vi "SISE-Monitor100-Demo.vi"() -> ()   [LabVIEW 2024]
uses:
  SubVIs-SISE-Monitor100/Control-IonFlux.ctl
  <vilib>/DAQmx/create/channels.llb/DAQmx Create Channel (AI-Voltage-Basic).vi
  <vilib>/Instr/_visa.llb/VISA Configure Serial Port (Instr).vi
  <vilib>/Analysis/NI_AALPro.lvlib
  <vilib>/DAQmx/read.llb/DAQmx Read (Analog 2D DBL NChan NSamp).vi
panel:
  out "Lesepuffer":string
  out "Registerkarte":enum32{"Start", "Record", "Stop"}(tab)
  out "Output V ch 2":bool
  in  "V channel 2":bool
  out "Output V ch 1":bool
  in  "V channel 1":bool
  out "SISE channel 1":bool
  out "Output SISE ch 2":bool
  in  "SISE channel 2":bool
  out "slow":bool
  in  "Scan angle (degrees)":dbl(slide) scale=0.0..90.0
  out "?":dbl
  in  "VISA res. name":refnum<visa-resource-name> caption="VISA-Ressourcenname"
  in  "Start measurement":bool
  out "Data File":bool
  out "Ind. Channel In":bool
  in  "Data file":path
  out "Ind. Channel Out":bool
  out "?":dbl
  out "Record period (round at 5s)":dbl
  in  "Scan distance (µm)":dbl(slide)=50.0 scale=0.0..100.0
  in  "Record period (single track, s)":dbl(slide)=10.112359550561797 scale=0.0..60.0 scale format="%#_2f"
  in  "Manipulator Speed":bool
  out "fast":bool
  in  "Channels In":tag
  in  "Position of manipulator":bool
  out "left":bool
  out "right":bool
  in  "TC 3":T1(tab)
  in  "Range limit\nS1.1 (mV)":dbl(slide)=200.0 min=0.0 max=600.0 scale=0.2..600.0
  in  "Base line\nS1.1 (mV)":dbl(slide) scale=-300.0..300.0
  in  "Range limit\nS1.2 mV":dbl(slide)=30.0 scale=0.1..30.0
  in  "Base line \nS1.2 (mV)":dbl(slide) scale=-15.0..15.0
  out "dV-SISE channel 1":cluster{dbl[], dbl[]}[](graph)
  out "V-SISE channel 1":cluster{dbl[], dbl[]}[](graph)
  out "V-SISE channel 2":cluster{dbl[], dbl[]}[](graph)
  out "dV-SISE channel 2":cluster{dbl[], dbl[]}[](graph)
  in  "Range limit\nS2.1 (mV)":dbl(slide)=200.0 min=0.0 max=600.0 scale=0.2..600.0
  in  "Base line\nS2.1 (mV)":dbl(slide) scale=-300.0..300.0
  in  "Base line \nS2.2 (mV)":dbl(slide) scale=-15.0..15.0
  in  "Range limit\nS2.2 (mV)":dbl(slide)=30.0 scale=0.1..30.0
  out "Voltage channel 1":cluster{dbl[], dbl[]}[](graph)
  in  "Base line\nV1 (V)":dbl(slide) scale=-300.0..300.0
  in  "Range limit\nV1 (V)":dbl(slide)=200.0 min=0.0 max=600.0 scale=0.2..600.0
  in  "Base line\nV2 (V)":dbl(slide) scale=-300.0..300.0
  in  "Range limit\nV2 (V)":dbl(slide)=200.0 min=0.0 max=600.0 scale=0.2..600.0
  out "Voltage channel 2":cluster{dbl[], dbl[]}[](graph)
  out "V channel #2":bool
  out "V channel #1":bool
  out "SISE channel #2":bool
  out "SISE channel #1":bool
  in  "?":T2(tab)
  in  "V SISE\nch #1":dbl(slide)=4.96774193548387 scale=-10.0..10.0
  out "Vprobe SISE 1":cluster{dbl[], dbl[]}[](graph)
  in  "V SISE\nch #2":dbl(slide)=4.96774193548387 scale=-10.0..10.0
  out "Vprobe SISE 2":cluster{dbl[], dbl[]}[](graph)
  in  "Vch #1":dbl(slide)=5.096774193548386 scale=-10.0..10.0
  out "Vprobe V 1":cluster{dbl[], dbl[]}[](graph)
  in  "Vch\n#2":dbl(slide)=5.096774193548386 scale=-10.0..10.0
  out "Vprobe V 2":cluster{dbl[], dbl[]}[](graph)
  in  "Enable change position 0":bool
  out "Raw data file":path
  in  "Stop measurent":bool
  out "Position probe":cluster{dbl[], dbl[]}[](graph)
  in  "Add Mark":bool
  in  "Event Mark":string
  out "Stop recording":bool
  out "String":string
  out "E-mark on":T3
  out "?":string
  in  "Bildlaufleiste":i32(c297)
  in  "Start fit (% of rec. period)":dbl(slide)=50.0 scale=0.0..100.0
  in  "?":enum32{"dV SISE 1", "dV SISE 2"}(tab)
  out "deltaV SISE 1":cluster{dbl[], "Best Linear Fit":dbl[]}[](graph)
  out "deltaV SISE 2":cluster{dbl[], "Best Linear Fit":dbl[]}[](graph)
  in  "Zoom from start":dbl(slide) scale=0.0..100.0
  in  "Zoom from end":dbl(slide)=100.0 scale=0.0..100.0
  in  "Stop programm":bool
  in  "New measurement":bool
  out "Stop recording 2":bool
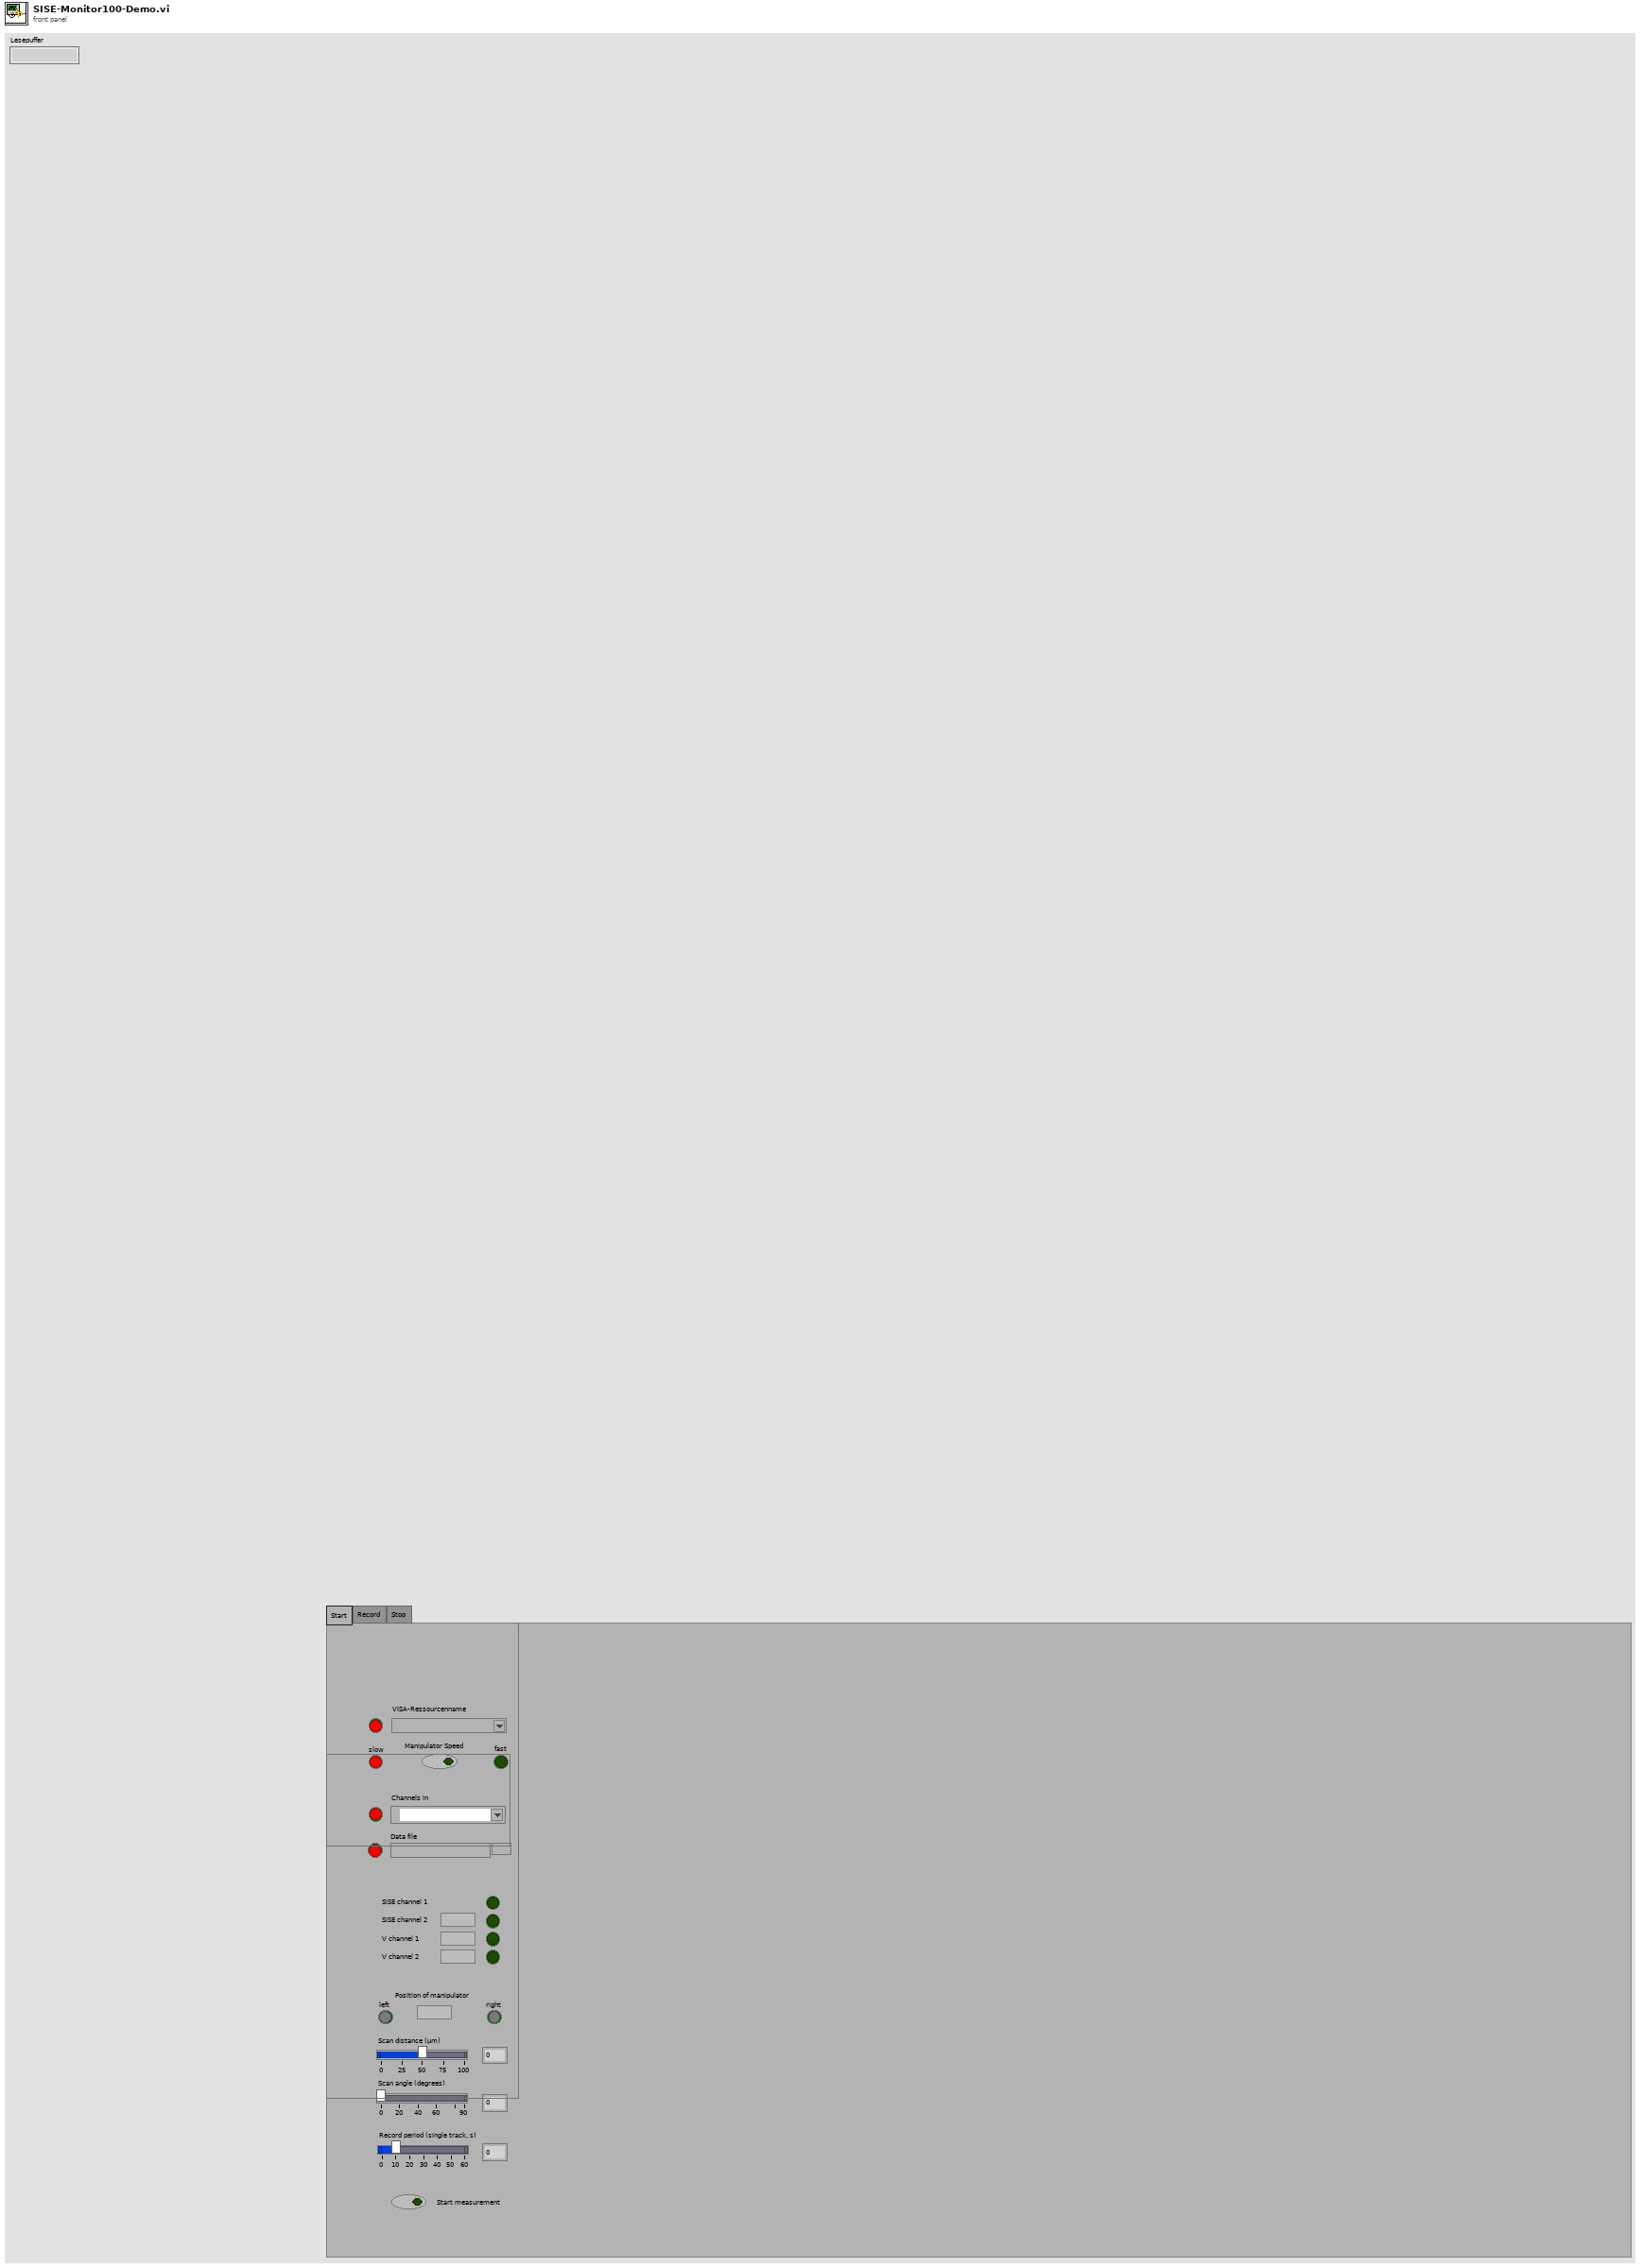
[diagram p1: front panel]
types:
  T1 = enum32{"SISE channel #1", "SISE channel #2", "V channel #1", "V channel #2"}
  T2 = enum32{"SISE chan #1", "SISE chan #2", "V chan #1", "V chan #2"}
  T3 = typedef "Control-IonFlux.ctl" = bool
  T4 = cluster{"refnum out":refnum<file>, "status":bool, "code":i32, "source":string}
  T5 = cluster{"task out":refnum<k21>, "status":bool, "code":i32, "source":string}
  T6 = enum16{"open", "replace", "create", "open or create", "replace or create", "replace or create with confirmation"}
  T7 = cluster{"refnum":refnum<file>, "status":bool, "code":i32, "source":string}
  T8 = cluster{dbl[], dbl[], "Best Linear Fit":dbl[], dbl[], dbl[]}
  T9 = cluster{"Array (Ausgang)":dbl[], "Array (Ausgang)":dbl[]}
  T10 = cluster{"Array (Ausgang)":dbl[], "Array (Ausgang)":dbl[]}[]
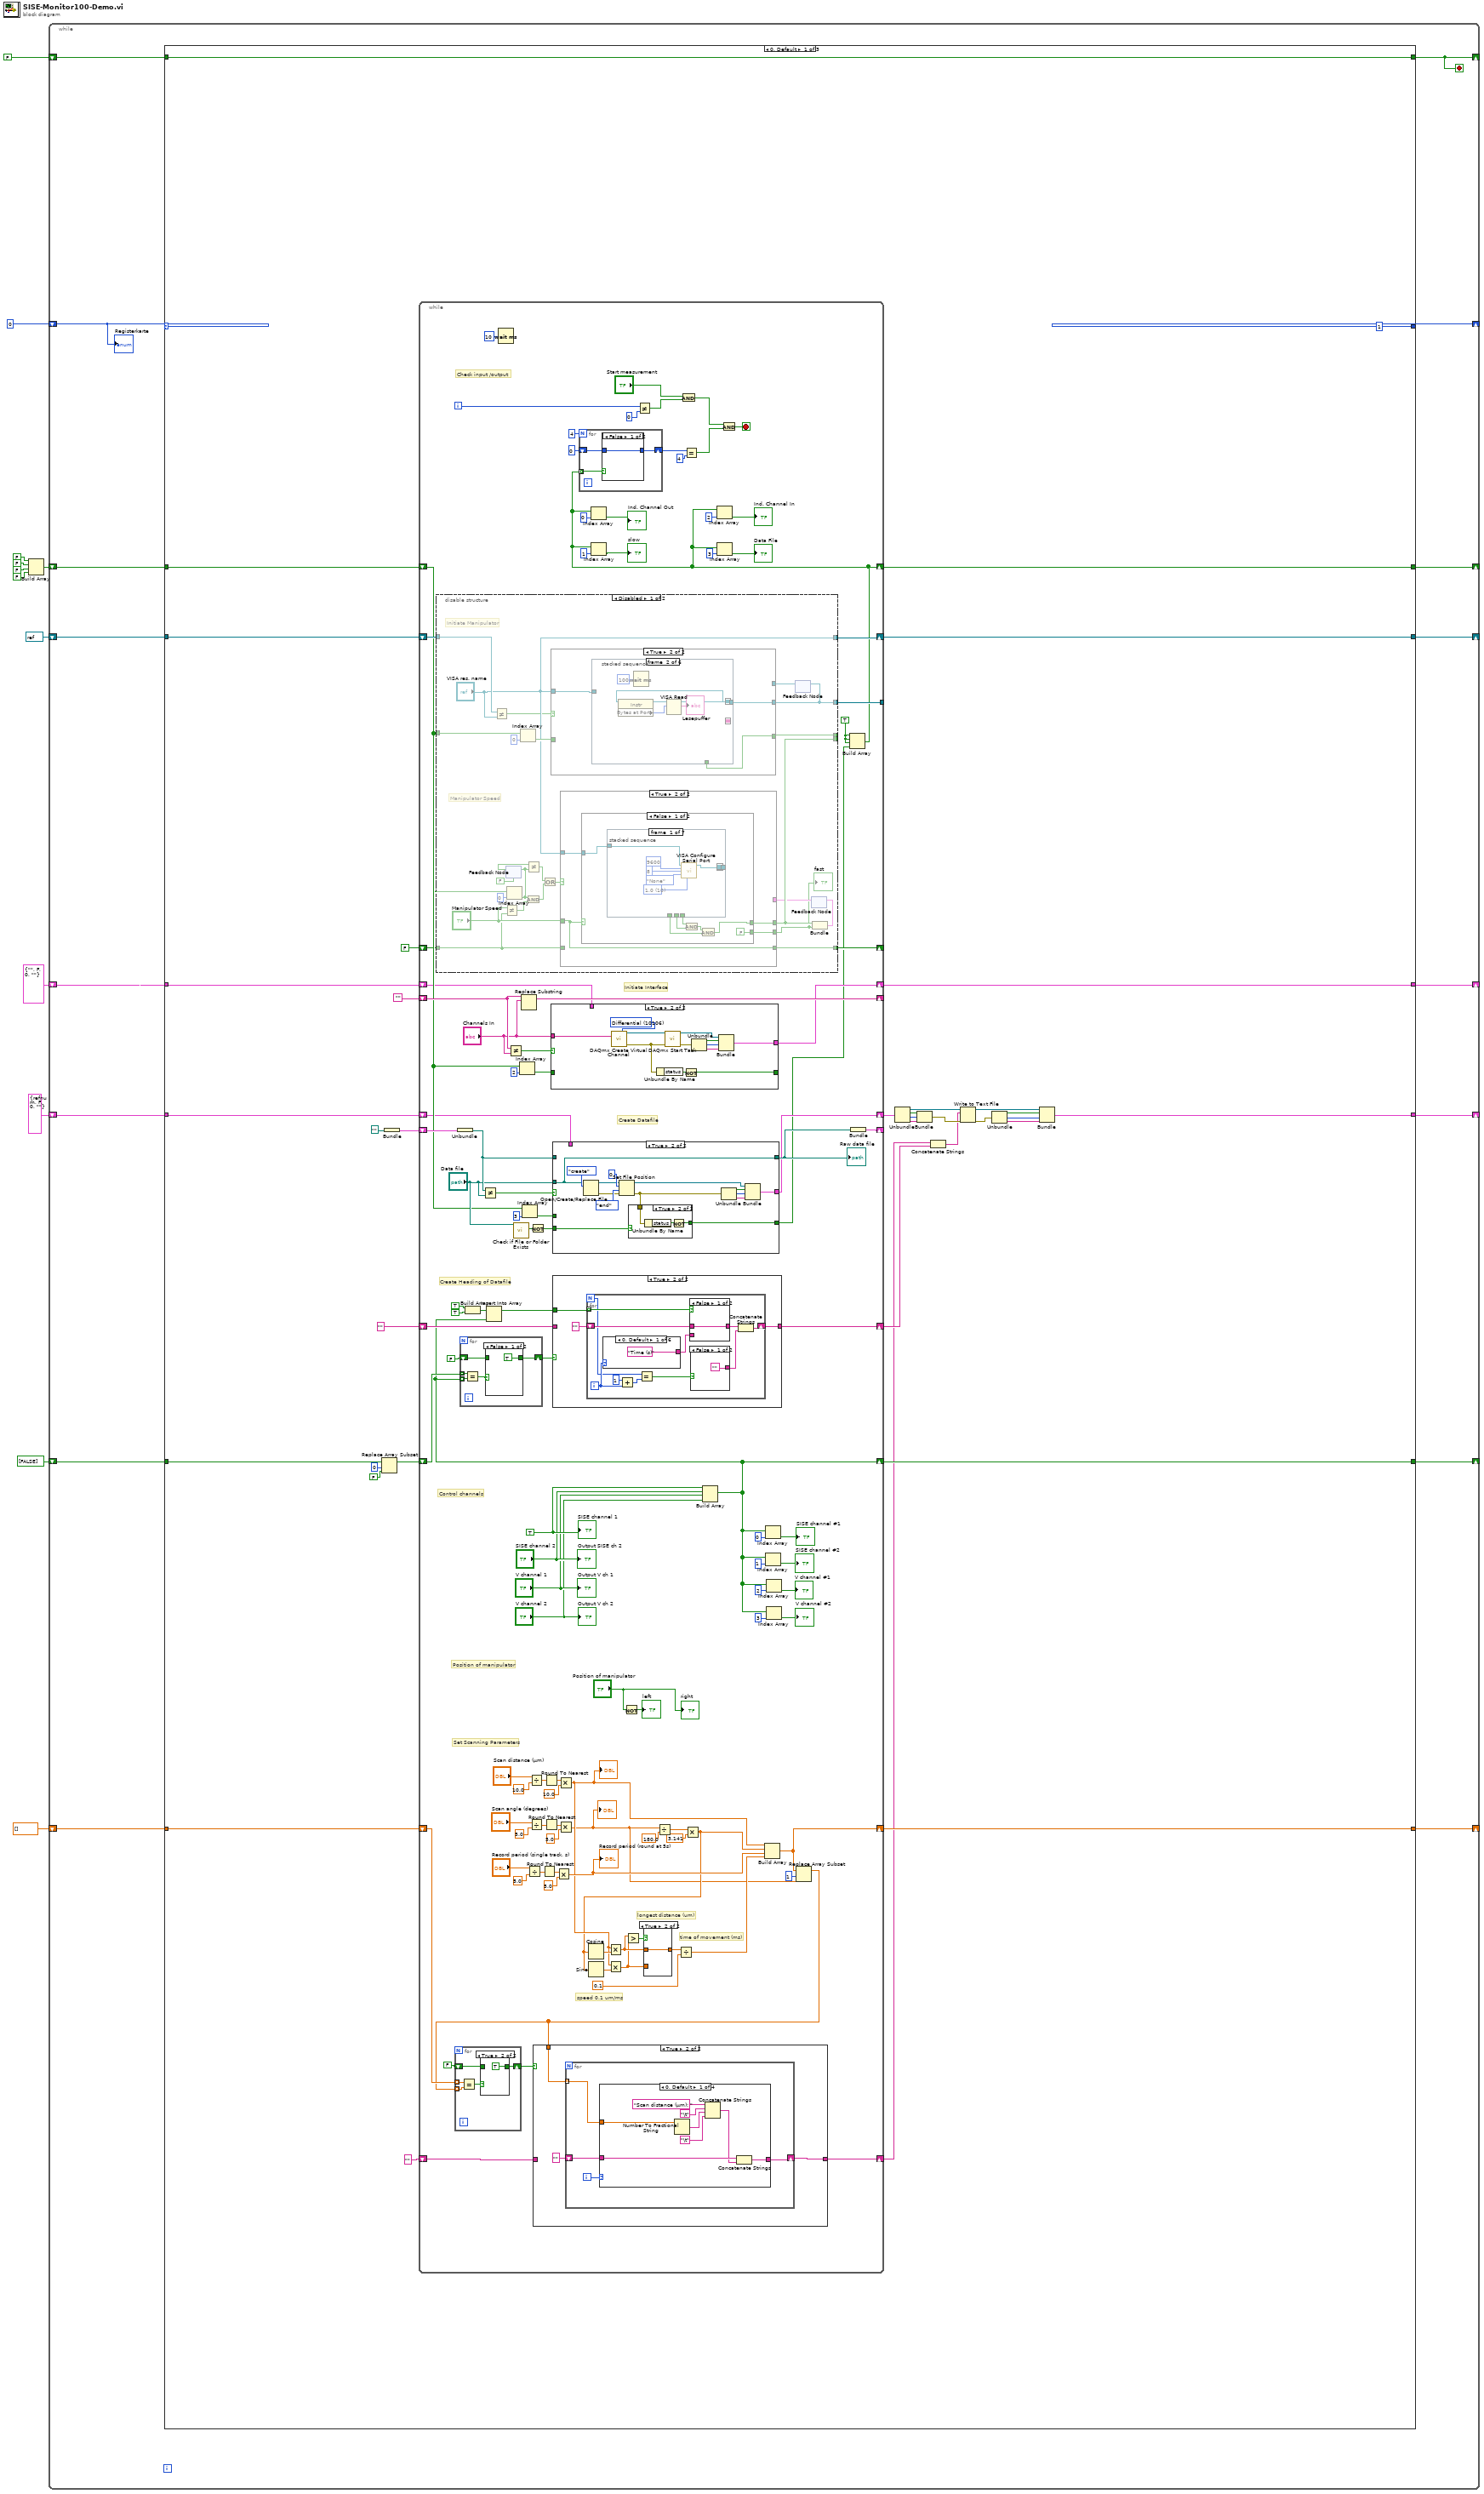
[diagram p0: block diagram]
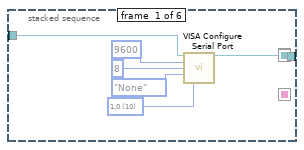
[diagram p3: hidden frame]
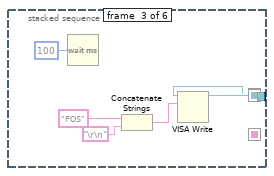
[diagram p4: hidden frame]
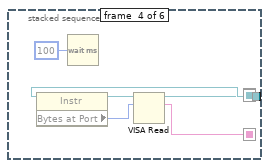
[diagram p5: hidden frame]
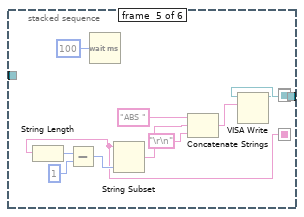
[diagram p6: hidden frame]
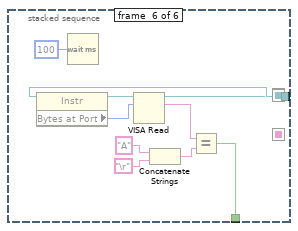
[diagram p7: hidden frame]
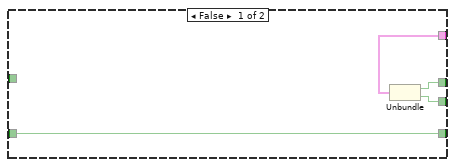
[diagram p8: hidden frame]
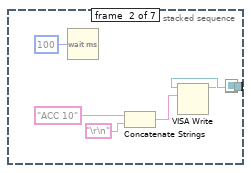
[diagram p9: hidden frame]
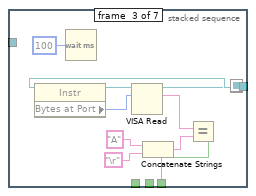
[diagram p10: hidden frame]
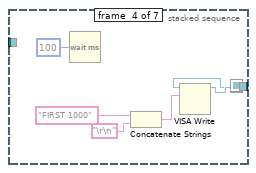
[diagram p11: hidden frame]
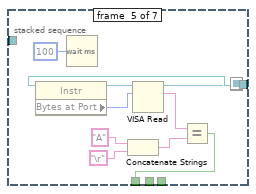
[diagram p12: hidden frame]
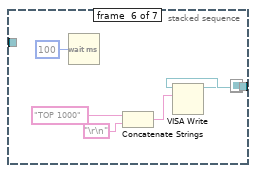
[diagram p13: hidden frame]
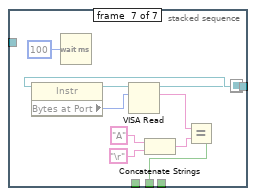
[diagram p14: hidden frame]
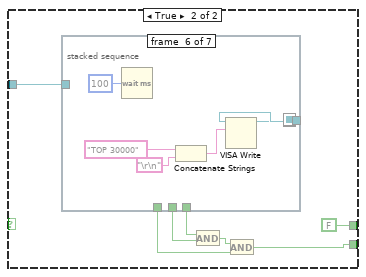
[diagram p15: hidden frame]
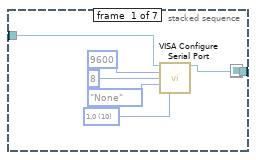
[diagram p16: hidden frame]
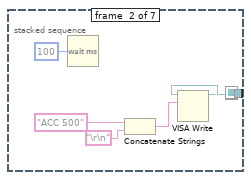
[diagram p17: hidden frame]
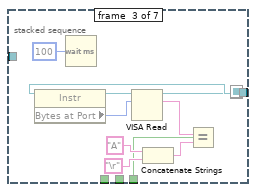
[diagram p18: hidden frame]
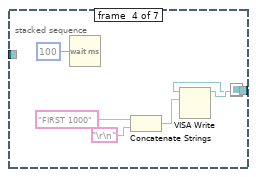
[diagram p19: hidden frame]
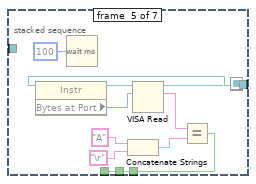
[diagram p20: hidden frame]
diagram:
  n1 = Build Array(FALSE, FALSE, FALSE, FALSE) -> (w1:bool[])
  n2 = while {
    shift-right: [w28] -> _
    shift-left: 0 -> [w27]
    shift-right: [w25] -> _
    shift-left: refnum<visa-resource-name> refnum ("VISA res. name") -> [w26]
    shift-right: [w23] -> _
    shift-left: T5 {"task out"="", "status"=FALSE, "code"=0, "source"=""} -> [w24]
    shift-right: [w19] -> _
    shift-left: T4 {"refnum out"=refnum, "status"=FALSE, "code"=0, "source"=""} -> [w20]
    shift-right: [w22] -> _
    shift-left: dbl[] [] -> [w21]
    shift-right: [w18] -> _
    shift-left: bool[] [FALSE] -> [w17]
    shift-right: [w15] -> _
    shift-left: FALSE -> [w16]
    shift-right: [w13] -> _
    shift-left: w1 -> [w14]
    stop <- w15 stop-if-true
    n3 = case shown="0, Default" w27 {
      tunnel: [1 2 0] -> w28
      tunnel: w26 -> [w60 w559 w1622]
      tunnel: [w59 w558 w1622] -> w25
      tunnel: w24 -> [w58 w557 w1621]
      tunnel: [w57 w553 w1621] -> w23
      tunnel: [w40 w532 w1619] -> w19
      tunnel: w20 -> [w56 w536 w1619]
      tunnel: [w55 w546 w1620] -> w22
      tunnel: w21 -> [w54 w546 w1620]
      tunnel: w17 -> [w31 w522 w1618]
      tunnel: [w53 w529 w1618] -> w18
      tunnel: w16 -> [w39 w521 w1617]
      tunnel: [w39 w521 w1616] -> w15
      tunnel: w14 -> [w33 w520 w1615]
      tunnel: [w38 w520 w1615] -> w13
      frame 0, Default {
        n4 = Replace Array Subset(array=w31, new element=FALSE ("Neues Element/Teil-Array"), index=0 ("Index")) -> (w32:bool[])
        n5 = Bundle(path "") -> (w61:cluster{path})  [unwired: 1 in]
        n6 = while {
          shift-right: [w117] -> w59
          shift-left: w60 -> [w165]
          shift-right: [w90] -> w38
          shift-left: w33 -> [w123]
          tunnel: [w124] -> _
          shift-right: [w160] -> _
          shift-left: "" -> [w159]
          shift-right: [w151] -> _
          shift-left: w61 -> [w153]
          shift-right: [w118] -> _
          shift-left: FALSE -> [w122]
          shift-right: [w115] -> w57
          shift-left: w58 -> [w116]
          shift-right: [w113] -> w51
          shift-left: w56 -> [w112]
          shift-right: [w73] -> w55
          shift-left: w54 -> [w77]
          shift-right: [w82] -> w53
          shift-left: w32 -> [w85]
          shift-right: [w87] -> w36
          shift-left: "" -> [w86]
          shift-right: [w79] -> w35
          shift-left: "" -> [w75]
          i -> [w80]
          stop <- w83 stop-if-true
          w68 = TRUE
          w108 = TRUE
          # "Position of manipulator"
          # "Set Scanning Parameters"
          # "Control channels"
          # "Create Heading of Datafile"
          # "Create Datafile"
          # "Initiate Interface"
          # "Check input /output"
          # "speed 0.1 um/ms"
          # "longest distance (um)"
          # "time of movement (ms)"
          n7 = disable-structure shown="Disabled" {
            disable-tunnel: w165 -> [w200 _]
            disable-tunnel: [w196 _] -> w124
            disable-tunnel: w123 -> [w194 _]
            disable-tunnel: w122 -> [w191 _]
            disable-tunnel: [w184 _] -> _
            disable-tunnel: [w183 _] -> _
            disable-tunnel: [w180 _] -> w118
            disable-tunnel: ["VISA res. name" _] -> w117
            frame Disabled {
              # "Manipulator Speed"
              # "Initiate Manipulator"
              n8 = Not Equal?(x=w200, y="VISA res. name") -> (x != y?=w177:bool)
              n9 = Not Equal?(x="Manipulator Speed", y=w191) -> (x != y?=w193:bool)
              n10 = feedback #1(FALSE) -> (w188:bool)
              n11 = Index Array(array=w194, index=0 ("Index")) -> (element=w189:bool)
              n12 = feedback-in #1(w189) -> ()
              n13 = Index Array(array=w194, index=0 ("Index")) -> (element=w198:bool)
              n14 = Not Equal?(x=w188, y=w189) -> (x != y?=w187:bool)
              n15 = And(x=w189, y=w193) -> (x .and. y?=w185:bool)
              n16 = Or(x=w187, y=w185) -> (x .or. y?=w186:bool)
              n17 = feedback #2() -> (w197:refnum<visa-resource-name>)  [unwired: 1 in]
              n18 = case shown="True" w177 {
                tunnel: w198 -> [w202 _]
                tunnel: [w202 w205] -> w184
                tunnel: "VISA res. name" -> [_ w204]
                tunnel: [w201 w203] -> w196
                tunnel: w197 -> [w201 _]
                frame False {
                }
                frame True {
                  n19 = stacked-sequence {
                    seq-local: [w206 _ _ _ _ _] -> [_ w213 _ _ _ _]
                    seq-local: [_ w214 _ _ _ _] -> [_ _ w218 _ _ _]
                    seq-local: [_ _ w219 _ _ _] -> [_ _ _ w226 _ _]
                    seq-local: [_ _ _ w225 _ _] -> [_ _ _ _ w237 _]
                    seq-local: [_ _ _ w224 _ _] -> [_ _ _ _ w231 _]
                    seq-local: [_ _ _ _ w236 _] -> [_ _ _ _ _ w247]
                    tunnel: w204 -> [w211 _ _ _ _ _]
                    tunnel: [_ _ _ _ _ w246] -> w203
                    tunnel: [_ _ _ _ _ w241] -> w205
                    frame #0 {
                      w207 = u16 10 items=["1,0"=10, "1,5"=15, "2,0"=20] ("stop bits (10: 1 bit)")
                      n20 = call-poly "VISA Configure Serial Port"("VISA resource name"=w211, "baud rate (9600)"=u32 9600, "data bits (8)"=u16 8, "parity (0:none)"=enum16{"None", "Odd", "Even", "Mark", "Space"}."None", "stop bits (10: 1 bit)"=w207) -> ("VISA resource name out"=w206:refnum<visa-resource-name>)  [unwired: 9 in, 1 out]
                    }
                    frame #1 {
                      n21 = property class="Instr"(reference=w213) -> (reference out=w216:refnum<visa-resource-name>, "Bytes at Port"=w215:u32)  [unwired: 1 in, 1 out]
                      n22 = Wait (ms)(milliseconds to wait=u32 100) -> ()  [unwired: 1 out]
                      n23 = VISA Read(VISA resource name=w216, byte count=w215) -> (VISA resource name out=w214:refnum<visa-resource-name>, read buffer=→"Lesepuffer":string)  [unwired: 1 in, 2 out]
                    }
                    frame #2 {
                      n24 = Wait (ms)(milliseconds to wait=u32 100) -> ()  [unwired: 1 out]
                      n25 = Concatenate Strings("POS", "\r\n") -> (w220:string)
                      n26 = VISA Write(VISA resource name=w218, write buffer=w220) -> (VISA resource name out=w219:refnum<visa-resource-name>)  [unwired: 1 in, 2 out]
                    }
                    frame #3 {
                      n27 = property class="Instr"(reference=w226) -> (reference out=w227:refnum<visa-resource-name>, "Bytes at Port"=w228:u32)  [unwired: 1 in, 1 out]
                      n28 = Wait (ms)(milliseconds to wait=u32 100) -> ()  [unwired: 1 out]
                      n29 = VISA Read(VISA resource name=w227, byte count=w228) -> (VISA resource name out=w225:refnum<visa-resource-name>, read buffer=w224:string)  [unwired: 1 in, 2 out]
                    }
                    frame #4 {
                      n30 = String Length(string=w231) -> (length=w234:i32)
                      n31 = Subtract(x=w234, y=1) -> (x-y=w232:i32)
                      n32 = Wait (ms)(milliseconds to wait=u32 100) -> ()  [unwired: 1 out]
                      n33 = String Subset(string=w231, length (rest)=w232) -> (substring=w230:string)  [unwired: 1 in]
                      n34 = Concatenate Strings("ABS ", w230, "\r\n") -> (w238:string)
                      n35 = VISA Write(VISA resource name=w237, write buffer=w238) -> (VISA resource name out=w236:refnum<visa-resource-name>)  [unwired: 1 in, 2 out]
                    }
                    frame #5 {
                      n36 = property class="Instr"(reference=w247) -> (reference out=w248:refnum<visa-resource-name>, "Bytes at Port"=w249:u32)  [unwired: 1 in, 1 out]
                      n37 = Wait (ms)(milliseconds to wait=u32 100) -> ()  [unwired: 1 out]
                      n38 = VISA Read(VISA resource name=w248, byte count=w249) -> (VISA resource name out=w246:refnum<visa-resource-name>, read buffer=w242:string)  [unwired: 1 in, 2 out]
                      n39 = Concatenate Strings("A", "\r") -> (w245:string)
                      n40 = Equal?(x=w242, y=w245) -> (x = y?=w241:bool)
                    }
                  }
                }
              }
              n41 = feedback-in #2(w196) -> ()
              n42 = feedback #3() -> (w181:cluster{bool, bool})  [unwired: 1 in]
              n43 = case shown="True" w186 {
                tunnel: "VISA res. name" -> [_ w258]
                tunnel: [w254 w257] -> w180
                tunnel: "Manipulator Speed" -> [_ w257]
                tunnel: w191 -> [w254 _]
                tunnel: [w251 w256] -> w183
                tunnel: [w252 w255] -> w178
                tunnel: w181 -> [w253 _]
                frame False {
                  n44 = Unbundle(w253) -> (w251:bool, w252:bool)
                }
                frame True {
                  n45 = case shown="False" w257 {
                    tunnel: w258 -> [w265 w326]
                    tunnel: [FALSE w320] -> w255
                    tunnel: [w259 FALSE] -> w256
                    frame False {
                      n46 = stacked-sequence {
                        seq-local: [w266 _ _ _ _ _ _] -> [_ w276 _ _ _ _ _]
                        seq-local: [_ w272 _ _ _ _ _] -> [_ _ w285 _ _ _ _]
                        seq-local: [_ _ w279 _ _ _ _] -> [_ _ _ w288 _ _ _]
                        seq-local: [_ _ _ w289 _ _ _] -> [_ _ _ _ w300 _ _]
                        seq-local: [_ _ _ _ w299 _ _] -> [_ _ _ _ _ w305 _]
                        seq-local: [_ _ _ _ _ w304 _] -> [_ _ _ _ _ _ w316]
                        tunnel: w265 -> [w271 _ _ _ _ _ _]
                        tunnel: [_ _ w278 _ _ _ _] -> w263
                        tunnel: [_ _ _ _ w294 _ _] -> w261
                        tunnel: [_ _ _ _ _ _ w315] -> _
                        tunnel: [_ _ _ _ _ _ w310] -> w262
                        frame #0 {
                          w267 = u16 10 items=["1,0"=10, "1,5"=15, "2,0"=20] ("stop bits (10: 1 bit)")
                          n47 = call-poly "VISA Configure Serial Port"("VISA resource name"=w271, "baud rate (9600)"=u32 9600, "data bits (8)"=u16 8, "parity (0:none)"=enum16{"None", "Odd", "Even", "Mark", "Space"}."None", "stop bits (10: 1 bit)"=w267) -> ("VISA resource name out"=w266:refnum<visa-resource-name>)  [unwired: 9 in, 1 out]
                        }
                        frame #1 {
                          n48 = Wait (ms)(milliseconds to wait=u32 100) -> ()  [unwired: 1 out]
                          n49 = Concatenate Strings("ACC 10", "\r\n") -> (w273:string)
                          n50 = VISA Write(VISA resource name=w276, write buffer=w273) -> (VISA resource name out=w272:refnum<visa-resource-name>)  [unwired: 1 in, 2 out]
                        }
                        frame #2 {
                          n51 = property class="Instr"(reference=w285) -> (reference out=w286:refnum<visa-resource-name>, "Bytes at Port"=w284:u32)  [unwired: 1 in, 1 out]
                          n52 = Wait (ms)(milliseconds to wait=u32 100) -> ()  [unwired: 1 out]
                          n53 = VISA Read(VISA resource name=w286, byte count=w284) -> (VISA resource name out=w279:refnum<visa-resource-name>, read buffer=w283:string)  [unwired: 1 in, 2 out]
                          n54 = Concatenate Strings("A", "\r") -> (w280:string)
                          n55 = Equal?(x=w283, y=w280) -> (x = y?=w278:bool)
                        }
                        frame #3 {
                          n56 = Wait (ms)(milliseconds to wait=u32 100) -> ()  [unwired: 1 out]
                          n57 = Concatenate Strings("FIRST 1000", "\r\n") -> (w290:string)
                          n58 = VISA Write(VISA resource name=w288, write buffer=w290) -> (VISA resource name out=w289:refnum<visa-resource-name>)  [unwired: 1 in, 2 out]
                        }
                        frame #4 {
                          n59 = property class="Instr"(reference=w300) -> (reference out=w301:refnum<visa-resource-name>, "Bytes at Port"=w302:u32)  [unwired: 1 in, 1 out]
                          n60 = Wait (ms)(milliseconds to wait=u32 100) -> ()  [unwired: 1 out]
                          n61 = Concatenate Strings("A", "\r") -> (w295:string)
                          n62 = VISA Read(VISA resource name=w301, byte count=w302) -> (VISA resource name out=w299:refnum<visa-resource-name>, read buffer=w298:string)  [unwired: 1 in, 2 out]
                          n63 = Equal?(x=w298, y=w295) -> (x = y?=w294:bool)
                        }
                        frame #5 {
                          n64 = Wait (ms)(milliseconds to wait=u32 100) -> ()  [unwired: 1 out]
                          n65 = Concatenate Strings("TOP 1000", "\r\n") -> (w306:string)
                          n66 = VISA Write(VISA resource name=w305, write buffer=w306) -> (VISA resource name out=w304:refnum<visa-resource-name>)  [unwired: 1 in, 2 out]
                        }
                        frame #6 {
                          n67 = property class="Instr"(reference=w316) -> (reference out=w317:refnum<visa-resource-name>, "Bytes at Port"=w318:u32)  [unwired: 1 in, 1 out]
                          n68 = Wait (ms)(milliseconds to wait=u32 100) -> ()  [unwired: 1 out]
                          n69 = VISA Read(VISA resource name=w317, byte count=w318) -> (VISA resource name out=w315:refnum<visa-resource-name>, read buffer=w311:string)  [unwired: 1 in, 2 out]
                          n70 = Concatenate Strings("A", "\r") -> (w314:string)
                          n71 = Equal?(x=w311, y=w314) -> (x = y?=w310:bool)
                        }
                      }
                      n72 = And(x=w263, y=w262) -> (x .and. y?=w264:bool)
                      n73 = And(x=w264, y=w261) -> (x .and. y?=w259:bool)
                    }
                    frame True {
                      n74 = stacked-sequence {
                        seq-local: [w327 _ _ _ _ _ _] -> [_ w337 _ _ _ _ _]
                        seq-local: [_ w333 _ _ _ _ _] -> [_ _ w346 _ _ _ _]
                        seq-local: [_ _ w340 _ _ _ _] -> [_ _ _ w349 _ _ _]
                        seq-local: [_ _ _ w350 _ _ _] -> [_ _ _ _ w361 _ _]
                        seq-local: [_ _ _ _ w360 _ _] -> [_ _ _ _ _ w366 _]
                        seq-local: [_ _ _ _ _ w365 _] -> [_ _ _ _ _ _ w377]
                        tunnel: w326 -> [w332 _ _ _ _ _ _]
                        tunnel: [_ _ w339 _ _ _ _] -> w324
                        tunnel: [_ _ _ _ w355 _ _] -> w322
                        tunnel: [_ _ _ _ _ _ w376] -> _
                        tunnel: [_ _ _ _ _ _ w371] -> w323
                        frame #0 {
                          w328 = u16 10 items=["1,0"=10, "1,5"=15, "2,0"=20] ("stop bits (10: 1 bit)")
                          n75 = call-poly "VISA Configure Serial Port"("VISA resource name"=w332, "baud rate (9600)"=u32 9600, "data bits (8)"=u16 8, "parity (0:none)"=enum16{"None", "Odd", "Even", "Mark", "Space"}."None", "stop bits (10: 1 bit)"=w328) -> ("VISA resource name out"=w327:refnum<visa-resource-name>)  [unwired: 9 in, 1 out]
                        }
                        frame #1 {
                          n76 = Wait (ms)(milliseconds to wait=u32 100) -> ()  [unwired: 1 out]
                          n77 = Concatenate Strings("ACC 500", "\r\n") -> (w334:string)
                          n78 = VISA Write(VISA resource name=w337, write buffer=w334) -> (VISA resource name out=w333:refnum<visa-resource-name>)  [unwired: 1 in, 2 out]
                        }
                        frame #2 {
                          n79 = property class="Instr"(reference=w346) -> (reference out=w347:refnum<visa-resource-name>, "Bytes at Port"=w345:u32)  [unwired: 1 in, 1 out]
                          n80 = Wait (ms)(milliseconds to wait=u32 100) -> ()  [unwired: 1 out]
                          n81 = VISA Read(VISA resource name=w347, byte count=w345) -> (VISA resource name out=w340:refnum<visa-resource-name>, read buffer=w344:string)  [unwired: 1 in, 2 out]
                          n82 = Concatenate Strings("A", "\r") -> (w341:string)
                          n83 = Equal?(x=w344, y=w341) -> (x = y?=w339:bool)
                        }
                        frame #3 {
                          n84 = Wait (ms)(milliseconds to wait=u32 100) -> ()  [unwired: 1 out]
                          n85 = Concatenate Strings("FIRST 1000", "\r\n") -> (w351:string)
                          n86 = VISA Write(VISA resource name=w349, write buffer=w351) -> (VISA resource name out=w350:refnum<visa-resource-name>)  [unwired: 1 in, 2 out]
                        }
                        frame #4 {
                          n87 = property class="Instr"(reference=w361) -> (reference out=w362:refnum<visa-resource-name>, "Bytes at Port"=w363:u32)  [unwired: 1 in, 1 out]
                          n88 = Wait (ms)(milliseconds to wait=u32 100) -> ()  [unwired: 1 out]
                          n89 = Concatenate Strings("A", "\r") -> (w356:string)
                          n90 = VISA Read(VISA resource name=w362, byte count=w363) -> (VISA resource name out=w360:refnum<visa-resource-name>, read buffer=w359:string)  [unwired: 1 in, 2 out]
                          n91 = Equal?(x=w359, y=w356) -> (x = y?=w355:bool)
                        }
                        frame #5 {
                          n92 = Wait (ms)(milliseconds to wait=u32 100) -> ()  [unwired: 1 out]
                          n93 = Concatenate Strings("TOP 30000", "\r\n") -> (w367:string)
                          n94 = VISA Write(VISA resource name=w366, write buffer=w367) -> (VISA resource name out=w365:refnum<visa-resource-name>)  [unwired: 1 in, 2 out]
                        }
                        frame #6 {
                          n95 = property class="Instr"(reference=w377) -> (reference out=w378:refnum<visa-resource-name>, "Bytes at Port"=w379:u32)  [unwired: 1 in, 1 out]
                          n96 = Wait (ms)(milliseconds to wait=u32 100) -> ()  [unwired: 1 out]
                          n97 = VISA Read(VISA resource name=w378, byte count=w379) -> (VISA resource name out=w376:refnum<visa-resource-name>, read buffer=w372:string)  [unwired: 1 in, 2 out]
                          n98 = Concatenate Strings("A", "\r") -> (w375:string)
                          n99 = Equal?(x=w372, y=w375) -> (x = y?=w371:bool)
                        }
                      }
                      n100 = And(x=w324, y=w323) -> (x .and. y?=w325:bool)
                      n101 = And(x=w325, y=w322) -> (x .and. y?=w320:bool)
                    }
                  }
                }
              }
              "fast" <- w178
              n102 = Bundle(w183, w178) -> (w182:cluster{bool, bool})  [unwired: 1 in]
              n103 = feedback-in #3(w182) -> ()
            }
            frame Enabled {
            }
          }
          n104 = Unbundle(w153) -> (w152:path)
          n105 = Build Array(TRUE, TRUE) -> (w93:bool[])
          n106 = Not Equal?(x=w152, y="Data file") -> (x != y?=w92:bool)
          n107 = Wait (ms)(milliseconds to wait=u32 10) -> ()  [unwired: 1 out]
          n108 = Not Equal?(x=w159, y="Channels In") -> (x != y?=w162:bool)
          n109 = call <vilib>:"Check if File or Folder Exists.vi"("path"="Data file") -> ("file or folder exists?"=w157:bool)  [unwired: 8 in, 2 out]
          n110 = Index Array(array=w123, index=2 ("Index")) -> (element=w161:bool)
          n111 = Replace Substring(4:"Channels In", 5:w159) -> (1:w160:string)  [unwired: 2 in, 1 out]
          n112 = Index Array(array=w123, index=3 ("Index")) -> (element=w154:bool)
          n113 = Divide(x="Record period (single track, s)", y=5.0) -> (x/y=w166:dbl)
          n114 = Divide(x="Scan distance (µm)", y=10.0) -> (x/y=w173:dbl)
          n115 = Divide(x="Scan angle (degrees)", y=5.0) -> (x/y=w141:dbl)
          n116 = Not(x=w157) -> (.not. x?=w149:bool)
          n117 = Round To Nearest(number=w166) -> (nearest integer value=w169:dbl)
          n118 = Round To Nearest(number=w173) -> (nearest integer value=w172:dbl)
          n119 = Round To Nearest(number=w141) -> (nearest integer value=w140:dbl)
          n120 = case shown="True" w162 {
            tunnel: w161 -> [w503 _]
            tunnel: [w503 w514] -> _
            tunnel: "Channels In" -> [_ w505]
            tunnel: w116 -> [w502 _]
            tunnel: [w502 w508] -> w115
            frame False {
            }
            frame True {
              w504 = 10106 items=["Default"=-1, "RSE"=10083, "NRSE"=10078, "Differential"=10106, "Pseudodifferential"=12529] ("input terminal configuration")
              n121 = call-poly <vilib>:"DAQmx Create Virtual Channel.vi"("input terminal configuration"=w504, "physical channels"=w505) -> ("task out"=w507:refnum<k21>, "error out"=w506:errorcluster)  [unwired: 12 in]
              n122 = Unbundle By Name(w506) -> ("status"=w515:bool)
              n123 = call <vilib>:"DAQmx Start Task.vi"("task/channels in"=w507, "error in"=w506) -> ("task out"=w509:refnum<k21>, "error out"=w513:errorcluster)  [unwired: 12 in]
              n124 = Not(x=w515) -> (.not. x?=w514:bool)
              n125 = Unbundle(w513) -> ("status"=w510:bool, "code"=w511:i32, "source"=w512:string)
              n126 = Bundle("task out"=w509, "status"=w510, "code"=w511, "source"=w512) -> (w508:T5)  [unwired: 1 in]
            }
          }
          n127 = case shown="True" w92 {
            tunnel: "Data file" -> [_ w491]
            tunnel: [w483 w492] -> w69
            tunnel: w154 -> [w483 _]
            tunnel: w152 -> [w482 _]
            tunnel: [w482 w491] -> w114
            tunnel: w149 -> [_ w490]
            tunnel: [w481 w486] -> w113
            tunnel: w112 -> [w481 _]
            frame False {
            }
            frame True {
              n128 = Open/Create/Replace File(file path (use dialog)=w491, operation (0:open)=T6."create") -> (refnum out=w495:refnum<file>, error out=w494:errorcluster)  [unwired: 4 in, 1 out]
              n129 = Set File Position(offset (in bytes) (0)=i64 0, refnum=w495, from (0:start)=enum16{"start", "end", "current"}."end", error in=w494) -> (refnum out=w484:refnum<file>, error out=w485:errorcluster)
              n130 = case shown="True" w490 {
                tunnel: [FALSE w500] -> w492
                tunnel: w485 -> [_ w499]
                frame False {
                }
                frame True {
                  n131 = Unbundle By Name(w499) -> ("status"=w501:bool)
                  n132 = Not(x=w501) -> (.not. x?=w500:bool)
                }
              }
              n133 = Unbundle(w485) -> ("status"=w489:bool, "code"=w488:i32, "source"=w487:string)
              n134 = Bundle("refnum"=w484, "status"=w489, "code"=w488, "source"=w487) -> (w486:T7)  [unwired: 1 in]
            }
          }
          "Raw data file" <- w114
          n135 = Multiply(x=w169, y=5.0) -> (x*y=w136:dbl)
          "Record period (round at 5s)" <- w136
          n136 = Multiply(x=w172, y=10.0) -> (x*y=w130:dbl)
          "?" <- w130
          n137 = Multiply(x=w140, y=5.0) -> (x*y=w71:dbl)
          "?" <- w71
          n138 = Not(x="Position of manipulator") -> (.not. x?=→"left":bool)
          n139 = Not Equal?(x=w80, y=0) -> (x != y?=w146:bool)
          n140 = Divide(x=w71, y=180.0) -> (x/y=w109:dbl)
          n141 = And(x="Start measurement", y=w146) -> (x .and. y?=w89:bool)
          n142 = Multiply(x=w109, y=3.141) -> (x*y=w74:dbl)
          n143 = Cosine(x=w74) -> (cos(x)=w135:dbl)
          n144 = Sine(x=w74) -> (sin(x)=w134:dbl)
          n145 = Multiply(x=w130, y=w135) -> (x*y=w133:dbl)
          n146 = Multiply(x=w130, y=w134) -> (x*y=w132:dbl)
          n147 = Greater?(x=w133, y=w132) -> (0:w131:bool)
          n148 = case shown="True" w131 {
            tunnel: w133 -> [_ w473]
            tunnel: w132 -> [w472 _]
            tunnel: [w472 w473] -> w129
            frame False {
            }
            frame True {
            }
          }
          n149 = Divide(x=w129, y=0.1) -> (x/y=w127:dbl)
          n150 = Build Array(w108, "SISE channel 2", "V channel 1", "V channel 2") -> (w82:bool[])
          n151 = for {
            tunnel: w85 -> [w432] mode=indexing
            tunnel: w82 -> [w431] mode=indexing
            shift-right: [w428] -> w81
            shift-left: FALSE -> [w429]
            n152 = Equal?(x=w432, y=w431) -> (x = y?=w430:bool)
            n153 = case shown="False" w430 {
              tunnel: w429 -> [_ w434]
              tunnel: [TRUE w434] -> w428
              frame False {
              }
              frame True {
              }
            }
          }
          n154 = Insert Into Array(array=w93, new element=w82) -> (w88:bool[])  [unwired: 1 in]
          n155 = case shown="True" w81 {
            tunnel: w88 -> [_ w437]
            tunnel: [w435 w436] -> w87
            tunnel: w86 -> [w435 _]
            frame False {
            }
            frame True {
              n156 = for {
                N -> [w441]
                shift-right: [w446] -> w436
                shift-left: "" -> [w449]
                tunnel: w437 -> [w447] mode=indexing
                i -> [w444]
                n157 = case shown="0, Default" w444 {
                  tunnel: ["Time (s)" w459 w462 w465 w468 w471] -> w448
                  frame 0, Default {
                  }
                  frame 1 {
                    n158 = Concatenate Strings("\t", "Position") -> (w459:string)
                  }
                  frame 2 {
                    n159 = Concatenate Strings("\t", "SISE 1 (mV)") -> (w462:string)
                  }
                  frame 3 {
                    n160 = Concatenate Strings("\t", "SISE 2 (mV)") -> (w465:string)
                  }
                  frame 4 {
                    n161 = Concatenate Strings("\t", "Voltage 1 (V)") -> (w468:string)
                  }
                  frame 5 {
                    n162 = Concatenate Strings("\t", "Voltage 2 (V)") -> (w471:string)
                  }
                }
                n163 = Add(x=1, y=w444) -> (x+y=w442:i32)
                n164 = Equal?(x=w441, y=w442) -> (x = y?=w440:bool)
                n165 = case shown="False" w447 {
                  tunnel: w449 -> [w452 w455]
                  tunnel: [w452 w454] -> w445
                  tunnel: w448 -> [_ w453]
                  frame False {
                  }
                  frame True {
                    n166 = Concatenate Strings(w455, w453) -> (w454:string)
                  }
                }
                n167 = case shown="False" w440 {
                  tunnel: ["" "\r\n"] -> w439
                  frame False {
                  }
                  frame True {
                  }
                }
                n168 = Concatenate Strings(w445, w439) -> (w446:string)
              }
            }
          }
          n169 = Build Array(w130, w74, w136, w127) -> (w73:dbl[])
          n170 = Index Array(array=w82, index=0 ("Index")) -> (element=→"SISE channel #1":bool)
          n171 = Index Array(array=w82, index=1 ("Index")) -> (element=→"SISE channel #2":bool)
          n172 = Index Array(array=w82, index=2 ("Index")) -> (element=→"V channel #1":bool)
          n173 = Index Array(array=w82, index=3 ("Index")) -> (element=→"V channel #2":bool)
          n174 = Replace Array Subset(array=w73, new element=w71, index=1 ("Index")) -> (w70:dbl[])
          n175 = for {
            shift-right: [w421] -> w76
            shift-left: FALSE -> [w422]
            tunnel: w77 -> [w425] mode=indexing
            tunnel: w70 -> [w424] mode=indexing
            n176 = Equal?(x=w425, y=w424) -> (x = y?=w423:bool)
            n177 = case shown="True" w423 {
              tunnel: w422 -> [w426 _]
              tunnel: [w426 TRUE] -> w421
              frame False {
              }
              frame True {
              }
            }
          }
          n178 = case shown="True" w76 {
            tunnel: [w381 w384] -> w79
            tunnel: w70 -> [_ w382]
            tunnel: w75 -> [w381 _]
            frame False {
            }
            frame True {
              n179 = for {
                tunnel: w382 -> [w385] mode=indexing
                shift-right: [w386] -> w384
                shift-left: "" -> [w387]
                i -> [w388]
                n180 = case shown="0, Default" w388 {
                  tunnel: [w396 w398 w408 w416] -> w386
                  tunnel: w387 -> [w395 w399 w407 w413]
                  tunnel: w385 -> [w391 w400 w406 w414]
                  frame 0, Default {
                    n181 = Number To Fractional String(number=w391) -> (F-format string=w390:string)  [unwired: 3 in]
                    n182 = Concatenate Strings("Scan distance (µm): ", "\t", w390, "\t") -> (w392:string)
                    n183 = Concatenate Strings(w395, w392) -> (w396:string)
                  }
                  frame 1 {
                    n184 = Number To Fractional String(number=w400) -> (F-format string=w404:string)  [unwired: 3 in]
                    n185 = Concatenate Strings("Scan angle (degrees): ", "\t", w404, "\t") -> (w397:string)
                    n186 = Concatenate Strings(w399, w397) -> (w398:string)
                  }
                  frame 2 {
                    n187 = Number To Fractional String(number=w406) -> (F-format string=w412:string)  [unwired: 3 in]
                    n188 = Concatenate Strings("Record period (single track, s): ", "\t", w412, "\t") -> (w405:string)
                    n189 = Concatenate Strings(w407, w405) -> (w408:string)
                  }
                  frame 3 {
                    n190 = Number To Fractional String(number=w414) -> (F-format string=w420:string)  [unwired: 3 in]
                    n191 = Concatenate Strings("Time of movement (ms): ", "\t", w420, "\r\n") -> (w415:string)
                    n192 = Concatenate Strings(w413, w415) -> (w416:string)
                  }
                }
              }
            }
          }
          n193 = Build Array(w68, w68, w68, w69) -> (w90:bool[])
          n194 = for {
            N: 4 -> [_]
            tunnel: w90 -> [w476] mode=indexing
            shift-right: [w474] -> w91
            shift-left: 0 -> [w475]
            n195 = case shown="False" w476 {
              tunnel: w475 -> [w477 w480]
              tunnel: [w477 w478] -> w474
              frame False {
              }
              frame True {
                n196 = Add(x=w480, y=1) -> (x+y=w478:i32)
              }
            }
          }
          n197 = Index Array(array=w90, index=0 ("Index")) -> (element=→"Ind. Channel Out":bool)
          n198 = Index Array(array=w90, index=1 ("Index")) -> (element=→"slow":bool)
          n199 = Equal?(x=w91, y=4) -> (x = y?=w142:bool)
          n200 = Index Array(array=w90, index=2 ("Index")) -> (element=→"Ind. Channel In":bool)
          n201 = Index Array(array=w90, index=3 ("Index")) -> (element=→"Data File":bool)
          n202 = And(x=w89, y=w142) -> (x .and. y?=w83:bool)
          n203 = Bundle("Data file"=w114) -> (w151:cluster{"Data file ":path})  [unwired: 1 in]
          "Output SISE ch 2" <- "SISE channel 2"
          "SISE channel 1" <- w108
          "Output V ch 1" <- "V channel 1"
          "Output V ch 2" <- "V channel 2"
          "right" <- "Position of manipulator"
        }
        n204 = Unbundle(w51) -> ("refnum out"=w46:refnum<file>, "status"=w50:bool, "code"=w49:i32, "source"=w48:string)
        n205 = Bundle("status"=w50, "code"=w49, "source"=w48) -> (w47:errorcluster)  [unwired: 1 in]
        n206 = Concatenate Strings(w35, w36) -> (w34:string)
        n207 = Write to Text File(file (use dialog)=w46, text=w34, error in=w47) -> (refnum out=w44:refnum<file>, error out=w45:errorcluster)  [unwired: 1 in, 1 out]
        n208 = Unbundle(w45) -> ("status"=w43:bool, "code"=w42:i32, "source"=w41:string)
        n209 = Bundle("refnum out"=w44, "status"=w43, "code"=w42, "source"=w41) -> (w40:T4)  [unwired: 1 in]
      }
      frame 1 {
        n210 = Index Array(array=w546, index=2 ("Index")) -> (element=w542:dbl)
        n211 = Build Array(0.0, 0.0, 0.0, 0.0, 0.0) -> (w523:dbl[])
        n212 = Multiply(x=w542, y=300.0 ("x")) -> (x*y=w547:dbl)
        n213 = Bundle(string[] [], dbl[][] []) -> (w539:cluster{string[], dbl[][]})  [unwired: 1 in]
        n214 = for {
          N: w547 -> [_]
          shift-right: [w569] -> w543
          shift-left: dbl[][] [] -> [w568]
          tunnel: w523 -> [w567]
          n215 = Insert Into Array(array=w568, new element=w567) -> (w569:dbl[][])  [unwired: 2 in]
        }
        n216 = Obtain Queue(element data type=w539) -> (queue out=w549:refnum<queue>, error out=w552:errorcluster)  [unwired: 4 in, 1 out]
        n217 = Get Date/Time In Seconds() -> (seconds since 1Jan1904=w565:timestamp)
        n218 = Build Array(0.0 ("Element"), 0.0 ("Element"), 0.0 ("Element")) -> (w560:dbl[])
        n219 = while {
          tunnel: w549 -> [w628]
          tunnel: w542 -> [w608]
          shift-right: [w580] -> _
          shift-left: w543 -> [w623]
          shift-right: [w597] -> _
          shift-left: dbl[][] [] -> [w598]
          shift-right: [w599] -> _
          shift-left: string[] ["Time, Event mark"] -> [w600]
          tunnel: w522 -> [w570]
          i -> [w579]
          stop <- w624 stop-if-true
          # "Replace time axis"
          # "Calculate average values"
          # "Determine dV"
          # "Combine traces for regression"
          n220 = local read "Stop recording"() -> (w625:bool)
          n221 = Dequeue Element(queue=w628) -> (element=w603:cluster{string[], dbl[][]}, error out=w627:errorcluster)  [unwired: 2 in, 2 out]
          n222 = local read "Start fit (% of rec. period)"() -> (w612:dbl)
          n223 = Greater Or Equal?(x=w579, y=2) -> (x >= y?=w590:bool)
          n224 = Unbundle By Name(w627) -> ("status"=w626:bool)
          n225 = Or(x=w626, y=w625) -> (x .or. y?=w624:bool)
          n226 = Unbundle(w603) -> (w601:string[], w602:dbl[][])
          n227 = Multiply(x=w608, y=w612) -> (x*y=w593:dbl)
          n228 = Multiply(x=w608, y=100.0) -> (x*y=w594:dbl)
          n229 = Multiply(x=w608, y=100.0) -> (x*y=w621:dbl)
          n230 = Multiply(x=w608, y=200.0) -> (x*y=w620:dbl)
          n231 = Array Subset(array=w623, index (row)=w621, length (row)=w620) -> (w617:dbl[][])  [unwired: 2 in]
          n232 = Delete From Array(array=w602, index (col)=1 ("Deaktivierter Index (Spalte)")) -> (array with subset deleted=w616:dbl[][])  [unwired: 2 in, 1 out]
          n233 = Insert Into Array(array=w617, new element=w616) -> (w580:dbl[][])  [unwired: 2 in]
          n234 = local read "Start fit (% of rec. period)"() -> (w609:dbl)
          n235 = Multiply(x=w608, y=w609) -> (x*y=w606:dbl)
          n236 = Multiply(x=w608, y=100.0) -> (x*y=w605:dbl)
          n237 = Add(x=w606, y=w605) -> (x+y=w607:dbl)
          n238 = Subtract(x=w605, y=w606) -> (x-y=w595:dbl)
          n239 = Array Subset(array=w580, index (row)=w607, length (row)=w595) -> (w582:dbl[][])  [unwired: 2 in]
          n240 = Transpose 2D Array(2D array=w582) -> (transposed array=w581:dbl[][])
          n241 = for {
            tunnel: w581 -> [w717] mode=indexing
            shift-right: [w716] -> w585
            shift-left: dbl[] [] -> [w715]
            n242 = Add Array Elements(numeric array=w717) -> (sum=w718:dbl)
            n243 = Array Size(array=w717) -> (size(s)=w719:i32)
            n244 = Divide(x=w718, y=w719) -> (x/y=w714:dbl)
            n245 = Insert Into Array(array=w715, new element=w714) -> (w716:dbl[])  [unwired: 1 in]
          }
          n246 = Index Array(array=w580, index (col)=0 ("Deaktivierter Index (Spalte)")) -> (element=w589:dbl[])  [unwired: 1 in]
          n247 = Index Array(array=w585, index=0 ("Index (Spalte)")) -> (element=w587:dbl)
          n248 = for {
            tunnel: w587 -> [w1058]
            shift-right: [w1061] -> w613
            shift-left: dbl[] [] -> [w1060]
            tunnel: w589 -> [w1057] mode=indexing
            n249 = Subtract(x=w1057, y=w1058) -> (x-y=w1059:dbl)
            n250 = Insert Into Array(array=w1060, new element=w1059) -> (w1061:dbl[])  [unwired: 1 in]
          }
          n251 = Replace Array Subset(array=w580, new element=w613, index (col)=0 ("Deaktivierter Index (Spalte)")) -> (w586:dbl[][])  [unwired: 1 in]
          n252 = for {
            N: 2 -> [_]
            tunnel: w586 -> [w644]
            tunnel: w594 -> [w643]
            tunnel: w593 -> [w642]
            tunnel: w590 -> [w638]
            tunnel: w579 -> [w636]
            shift-right: [w635] -> w583
            shift-left: dbl[] [] -> [w634]
            i -> [w641]
            n253 = flat-sequence {
              tunnel: w644 -> [w655]
              tunnel: w642 -> [w656]
              tunnel: w643 -> [w663]
              tunnel: [w660] -> w646
              tunnel: [w657] -> w645
              tunnel: w637 -> [w651]
              tunnel: w646 -> [w687]
              tunnel: w645 -> [w693]
              tunnel: w636 -> [w688]
              tunnel: [w676] -> w633
              tunnel: [w675] -> w639
              frame #0 {
                n254 = Subtract(x=w663, y=w656) -> (x-y=w669:dbl)
                n255 = Multiply(x=w663, y=2.0) -> (x*y=w666:dbl)
                n256 = Add(x=w656, y=w666) -> (x+y=w674:dbl)
                n257 = Add(x=w656, y=w663) -> (x+y=w673:dbl)
                n258 = Array Subset(array=w655, index (row)=w656, length (row)=w669) -> (w671:dbl[][])  [unwired: 2 in]
                n259 = Array Subset(array=w655, index (row)=w674, length (row)=w669) -> (w672:dbl[][])  [unwired: 2 in]
                n260 = Array Subset(array=w655, index (row)=w673, length (row)=w669) -> (w664:dbl[][])  [unwired: 2 in]
                n261 = Insert Into Array(array=w671, new element=w672) -> (w667:dbl[][])  [unwired: 2 in]
                n262 = Index Array(array=w664, index (col)=w651) -> (element=w654:dbl[])  [unwired: 1 in]
                n263 = Index Array(array=w667, index (col)=0 ("disabled index (col)")) -> (element=w662:dbl[])  [unwired: 1 in]
                n264 = Index Array(array=w664, index (col)=0 ("disabled index (col)")) -> (element=w653:dbl[])  [unwired: 1 in]
                n265 = Index Array(array=w667, index (col)=w651) -> (element=w661:dbl[])  [unwired: 1 in]
                n266 = call <vilib>:"Linear Fit.vi"("Y"=w661, "X"=w662) -> ("Best Linear Fit"=w652:dbl[], "slope"=w659:dbl, "intercept"=w658:dbl)  [unwired: 9 in, 2 out]
                n267 = Build Array(w659, w658) -> (w657:dbl[])
                n268 = Bundle(w662, w661, "Best Linear Fit"=w652, w653, w654) -> (w660:T8)  [unwired: 1 in]
              }
              frame #1 {
                n269 = Unbundle(w687) -> (w698:dbl[], w699:dbl[])  [unwired: 3 out]
                n270 = Divide(x=w688, y=2 ("x")) -> (x/y=w689:dbl)
                n271 = Index Array(array=w693, index=0 ("Index")) -> (element=w700:dbl)
                n272 = Index Array(array=w693, index=1 ("Index")) -> (element=w692:dbl)
                n273 = Unbundle(w687) -> (w684:dbl[], w686:dbl[], "Best Linear Fit"=w683:dbl[], w682:dbl[], w680:dbl[])
                n274 = Round To Nearest(number=w689) -> (nearest integer value=w690:dbl)
                n275 = Absolute Value(x=w700) -> (abs(x)=w705:dbl)
                n276 = Equal?(x=w690, y=w689) -> (x = y?=w695:bool)
                n277 = Divide(x=w705, y=1000.0) -> (x/y=w707:dbl)
                n278 = Bundle(w684, w686) -> (w685:cluster{dbl[], dbl[]})  [unwired: 1 in]
                n279 = Bundle(w684, "Best Linear Fit"=w683) -> (w679:cluster{dbl[], "Best Linear Fit":dbl[]})  [unwired: 1 in]
                n280 = Bundle(w682, w680) -> (w677:cluster{dbl[], dbl[]})  [unwired: 1 in]
                n281 = Subtract(x=w700, y=w707) -> (x-y=w704:dbl)
                n282 = Add(x=w700, y=w707) -> (x+y=w703:dbl)
                n283 = Bundle(w704, w703, -inf, inf) -> (w702:cluster{dbl, dbl, dbl, dbl})  [unwired: 1 in]
                n284 = call <vilib>:"Linear Fit.vi"("Y"=w699, "X"=w698, "parameter bounds"=w702) -> ("Best Linear Fit"=w681:dbl[], "intercept"=w691:dbl)  [unwired: 8 in, 3 out]
                n285 = Subtract(x=w692, y=w691) -> (x-y=w696:dbl)
                n286 = Bundle(w682, "Best Linear Fit"=w681) -> (w678:cluster{dbl[], "Best Linear Fit":dbl[]})  [unwired: 1 in]
                n287 = case shown="True" w695 {
                  tunnel: w696 -> [w710 w712]
                  tunnel: [w710 w713] -> w676
                  frame False {
                  }
                  frame True {
                    n288 = Multiply(x=-1.0, y=w712) -> (x*y=w713:dbl)
                  }
                }
                n289 = Build Array(w685, w679, w678, w677) -> (w675:cluster{dbl[], "Best Linear Fit":dbl[]}[])
              }
            }
            n290 = Add(x=1, y=w641) -> (x+y=w637:i32)
            n291 = case shown="True" w638 {
              tunnel: w639 -> [_ w648]
              tunnel: w637 -> [_ w647]
              frame False {
              }
              frame True {
                n292 = case shown="0, Default" w647 {
                  tunnel: w648 -> [_ w649 w650]
                  frame 0, Default {
                  }
                  frame 1 {
                    "deltaV SISE 1" <- w649
                  }
                  frame 2 {
                    "deltaV SISE 2" <- w650
                  }
                }
              }
            }
            n293 = Insert Into Array(array=w634, new element=w633) -> (w635:dbl[])  [unwired: 1 in]
          }
          n294 = Insert Into Array(array=w585, index=3 ("Index"), new element=w583) -> (w572:dbl[])
          n295 = Index Array(array=w572, index=0 ("Index")) -> (element=w574:dbl)
          n296 = Divide(x=w574, y=60.0) -> (x/y=w573:dbl)
          n297 = Replace Array Subset(array=w572, new element=w573, index=0 ("Index")) -> (w571:dbl[])
          n298 = case shown="True" w590 {
            tunnel: w598 -> [w629 w632]
            tunnel: [w629 w631] -> w597
            tunnel: w571 -> [_ w630]
            frame False {
            }
            frame True {
              n299 = Insert Into Array(array=w632, new element=w630) -> (w631:dbl[][])  [unwired: 2 in]
            }
          }
          n300 = while {
            tunnel: w597 -> [w726]
            tunnel: w601 -> [w743]
            tunnel: w600 -> [w742]
            tunnel: [w733] -> w599
            tunnel: w579 -> [w732]
            tunnel: w579 -> [w727]
            tunnel: w570 -> [w725]
            i -> [w777]
            stop <- w722 stop-if-true
            n301 = for {
              tunnel: w743 -> [w1037] mode=indexing
              shift-right: [w1034] -> w728
              shift-left: TRUE -> [w1038]
              n302 = Equal?(x=w1037, y="") -> (x = y?=w1035:bool)
              n303 = case shown="True" w1035 {
                tunnel: w1038 -> [_ w1040]
                tunnel: [FALSE w1040] -> w1034
                frame False {
                }
                frame True {
                }
              }
            }
            n304 = Wait (ms)(milliseconds to wait=u32 100 ("Zu wartende ms")) -> ()  [unwired: 1 out]
            n305 = Multiply(x="Zoom from end", y=-1.0) -> (x*y=w761:dbl)
            n306 = Add(x="Zoom from start", y=w761) -> (x+y=w772:dbl)
            n307 = feedback #4() -> (w767:dbl)  [unwired: 1 in]
            n308 = Greater Or Equal?(x=w772, y=0.0) -> (x >= y?=w770:bool)
            n309 = Less?(x=w732, y=2) -> (x < y?=w730:bool)
            n310 = case shown="True" w770 {
              tunnel: "Zoom from start" -> [w1049 w1052]
              tunnel: [w1048 w1052] -> w768
              tunnel: w767 -> [w1048 w1054]
              tunnel: "Zoom from end" -> [_ w1051]
              tunnel: [w1049 w1052] -> w760
              tunnel: [w1047 w1050] -> w759
              tunnel: "Zoom from end" -> [w1047 w1050]
              frame False {
              }
              frame True {
                n311 = Not Equal?(x=w1054, y=w1052) -> (x != y?=w1053:bool)
                n312 = case shown="False" w1053 {
                  tunnel: w1052 -> [_ w1056]
                  tunnel: w1051 -> [w1055 _]
                  frame False {
                    n313 = local write "Zoom from start"(w1055) -> ()
                  }
                  frame True {
                    n314 = local write "Zoom from end"(w1056) -> ()
                  }
                }
              }
            }
            n315 = feedback-in #4(w768) -> ()
            n316 = Or(x=w728, y=w730) -> (x .or. y?=w729:bool)
            n317 = case shown="False" w729 {
              tunnel: w742 -> [w1030 w1033]
              tunnel: [w1032 w1033] -> w733
              tunnel: w743 -> [w1031 _]
              frame False {
                n318 = Insert Into Array(array=w1030, new element=w1031) -> (w1032:string[])  [unwired: 1 in]
              }
              frame True {
              }
            }
            n319 = Array Size(array=w733) -> (size(s)=w739:i32)
            n320 = Array Subset(array=w733, index=1 ("Index")) -> (w747:string[])  [unwired: 1 in]
            n321 = Subtract(x=w759, y=w760) -> (x-y=w766:dbl)
            n322 = Divide(x=w739, y=10) -> (x/y=w737:dbl)
            n323 = for {
              tunnel: w747 -> [w1043] mode=indexing
              shift-right: [w1046] -> w745
              shift-left: dbl[] [] -> [w1045]
              n324 = Match Pattern(string=w1043, regular expression="\t") -> (before substring=w1041:string)  [unwired: 1 in, 3 out]
              n325 = Fract/Exp String To Number(string=w1041) -> (number=w1044:dbl)  [unwired: 3 in, 1 out]
              n326 = Insert Into Array(array=w1045, new element=w1044) -> (w1046:dbl[])  [unwired: 1 in]
            }
            n327 = Index Array(array=w726, index (col)=0 ("Deaktivierter Index (Spalte)")) -> (element=w774:dbl[])  [unwired: 1 in]
            n328 = Multiply(x=w737, y="Bildlaufleiste") -> (x*y=w735:dbl)
            n329 = Divide(x=w760, y=100.0) -> (x/y=w762:dbl)
            n330 = Divide(x=w766, y=100.0) -> (x/y=w763:dbl)
            n331 = Array Size(array=w774) -> (size(s)=w756:i32)
            n332 = Array Subset(array=w733, index=w735) -> (w734:string[])  [unwired: 1 in]
            n333 = Multiply(x=w756, y=w762) -> (x*y=w752:dbl)
            n334 = Multiply(x=w756, y=w763) -> (x*y=w755:dbl)
            n335 = Index Array(array=w725, index="TC 3") -> (element=w724:bool)
            n336 = Add(x=w755, y=2.0) -> (x+y=w753:dbl)
            n337 = Subtract(x=w752, y=2.0) -> (x-y=w750:dbl)
            n338 = for {
              shift-right: [w1028] -> w740
              shift-left: "" -> [w1029]
              tunnel: w734 -> [w1026] mode=indexing
              n339 = Concatenate Strings(w1029, w1026, "\r") -> (w1028:string)
            }
            "?" <- w740
            n340 = Array Subset(array=w726, index (row)=w750, length (row)=w753) -> (w746:dbl[][])  [unwired: 2 in]
            n341 = case shown="\"SISE channel #1\", Default" "TC 3" {
              tunnel: w746 -> [w789 w869 w981 w992]
              tunnel: w745 -> [w787 w868 w949 w995]
              tunnel: w727 -> [w786 w865 w946 w987]
              tunnel: w724 -> [w783 w864 w945 w986]
              frame "SISE channel #1", Default {
                n342 = Greater Or Equal?(x=w786, y=2) -> (x >= y?=w784:bool)
                n343 = And(x=w784, y=w783) -> (x .and. y?=w782:bool)
                n344 = Index Array(array=w789, index (col)=0 ("disabled index (col)")) -> (element=w792:dbl[])  [unwired: 1 in]
                n345 = Index Array(array=w789, index (col)=1 ("disabled index (col)")) -> (element=w791:dbl[])  [unwired: 1 in]
                n346 = Index Array(array=w789, index (col)=3 ("disabled index (col)")) -> (element=w788:dbl[])  [unwired: 1 in]
                n347 = stacked-sequence {
                  tunnel: w792 -> [w796 w835]
                  tunnel: w791 -> [w815 _]
                  tunnel: w787 -> [w797 w834]
                  tunnel: w788 -> [_ w833]
                  tunnel: w782 -> [w795 w829]
                  frame #0 {
                    n348 = Array Max & Min(array=w796) -> (max value=w807:dbl, min value=w806:dbl)  [unwired: 2 out]
                    n349 = Divide(x="Range limit\nS1.1 (mV)", y=2.0) -> (x/y=w825:dbl)
                    n350 = Divide(x="Range limit\nS1.1 (mV)", y=2.05) -> (x/y=w826:dbl)
                    n351 = Add(x="Base line\nS1.1 (mV)", y=w825) -> (x+y=w798:dbl)
                    n352 = Subtract(x="Base line\nS1.1 (mV)", y=w825) -> (x-y=w799:dbl)
                    n353 = Subtract(x="Base line\nS1.1 (mV)", y=w826) -> (x-y=w805:dbl)
                    n354 = call "EventstoGraph (SubVI).vi"("Numerisch 2"=w806, "Array 3"=w797, "Numerisch"=w807, "Array (Eingang)"=dbl[][] [], "Numerisch 3"=w805) -> ("Array (Ausgang)"=w809:dbl[][])  [unwired: 6 in]
                    n355 = Array Max & Min(array=w796) -> (max value=w821:dbl, min value=w822:dbl)  [unwired: 2 out]
                    n356 = call "GraphLimit01.vi"("Numeric 2"=w799, "Numeric"=w798, "Array in"=w815, "Array 3"=dbl[] []) -> ("Array out"=w814:dbl[])  [unwired: 7 in]
                    n357 = Build Array("Base line\nS1.1 (mV)", "Base line\nS1.1 (mV)") -> (w818:dbl[])
                    n358 = Build Array(w821, w822) -> (w819:dbl[])
                    n359 = Build Array(w798, w799) -> (w820:dbl[])
                    n360 = Index Array(array=w809, index (col)=0 ("Index (Zeile)")) -> (element=w810:dbl[])  [unwired: 1 in]
                    n361 = Index Array(array=w809, index (col)=1 ("Index (Zeile)")) -> (element=w808:dbl[])  [unwired: 1 in]
                    n362 = Bundle(w819, w820) -> (w802:cluster{dbl[], dbl[]})  [unwired: 1 in]
                    n363 = Bundle(w819, w818) -> (w803:cluster{dbl[], dbl[]})  [unwired: 1 in]
                    n364 = Bundle(w796, "Array out"=w814) -> (w801:cluster{dbl[], "Array out":dbl[]})  [unwired: 1 in]
                    n365 = Bundle("Array (Ausgang)"=w810, "Array (Ausgang)"=w808) -> (w800:T9)  [unwired: 1 in]
                    n366 = Build Array(w803, w802, w801, w800) -> (w804:T10)
                    n367 = case shown="True" w795 {
                      tunnel: w804 -> [_ w828]
                      frame False {
                      }
                      frame True {
                        "V-SISE channel 1" <- w828
                      }
                    }
                  }
                  frame #1 {
                    n368 = Array Max & Min(array=w835) -> (max value=w844:dbl, min value=w843:dbl)  [unwired: 2 out]
                    n369 = Divide(x="Range limit\nS1.2 mV", y=2.0) -> (x/y=w860:dbl)
                    n370 = Divide(x="Range limit\nS1.2 mV", y=2.05) -> (x/y=w861:dbl)
                    n371 = Add(x="Base line \nS1.2 (mV)", y=w860) -> (x+y=w836:dbl)
                    n372 = Subtract(x="Base line \nS1.2 (mV)", y=w860) -> (x-y=w837:dbl)
                    n373 = Subtract(x="Base line \nS1.2 (mV)", y=w861) -> (x-y=w842:dbl)
                    n374 = call "EventstoGraph (SubVI).vi"("Numerisch 2"=w843, "Array 3"=w834, "Numerisch"=w844, "Array (Eingang)"=dbl[][] [], "Numerisch 3"=w842) -> ("Array (Ausgang)"=w846:dbl[][])  [unwired: 6 in]
                    n375 = Array Max & Min(array=w835) -> (max value=w856:dbl, min value=w857:dbl)  [unwired: 2 out]
                    n376 = call "GraphLimit01.vi"("Numeric 2"=w837, "Numeric"=w836, "Array in"=w833, "Array 3"=dbl[] []) -> ("Array out"=w851:dbl[])  [unwired: 7 in]
                    n377 = Build Array("Base line \nS1.2 (mV)", "Base line \nS1.2 (mV)") -> (w853:dbl[])
                    n378 = Build Array(w856, w857) -> (w854:dbl[])
                    n379 = Build Array(w836, w837) -> (w855:dbl[])
                    n380 = Index Array(array=w846, index (col)=0 ("Index (Zeile)")) -> (element=w847:dbl[])  [unwired: 1 in]
                    n381 = Index Array(array=w846, index (col)=1 ("Index (Zeile)")) -> (element=w845:dbl[])  [unwired: 1 in]
                    n382 = Bundle(w854, w855) -> (w840:cluster{dbl[], dbl[]})  [unwired: 1 in]
                    n383 = Bundle(w854, w853) -> (w841:cluster{dbl[], dbl[]})  [unwired: 1 in]
                    n384 = Bundle(w835, "Array out"=w851) -> (w839:cluster{dbl[], "Array out":dbl[]})  [unwired: 1 in]
                    n385 = Bundle("Array (Ausgang)"=w847, "Array (Ausgang)"=w845) -> (w838:T9)  [unwired: 1 in]
                    n386 = Build Array(w841, w840, w839, w838) -> (w830:T10)
                    n387 = case shown="True" w829 {
                      tunnel: w830 -> [_ w862]
                      frame False {
                      }
                      frame True {
                        "dV-SISE channel 1" <- w862
                      }
                    }
                  }
                }
              }
              frame "SISE channel #2" {
                n388 = Greater Or Equal?(x=w865, y=2) -> (x >= y?=w867:bool)
                n389 = And(x=w867, y=w864) -> (x .and. y?=w863:bool)
                n390 = Index Array(array=w869, index (col)=0 ("disabled index (col)")) -> (element=w873:dbl[])  [unwired: 1 in]
                n391 = Index Array(array=w869, index (col)=2 ("disabled index (col)")) -> (element=w874:dbl[])  [unwired: 1 in]
                n392 = Index Array(array=w869, index (col)=4 ("disabled index (col)")) -> (element=w875:dbl[])  [unwired: 1 in]
                n393 = stacked-sequence {
                  tunnel: w873 -> [w877 w916]
                  tunnel: w874 -> [w896 _]
                  tunnel: w868 -> [w878 w915]
                  tunnel: w875 -> [_ w914]
                  tunnel: w863 -> [w876 w910]
                  frame #0 {
                    n394 = Array Max & Min(array=w877) -> (max value=w888:dbl, min value=w887:dbl)  [unwired: 2 out]
                    n395 = Divide(x="Range limit\nS2.1 (mV)", y=2.0) -> (x/y=w906:dbl)
                    n396 = Divide(x="Range limit\nS2.1 (mV)", y=2.05) -> (x/y=w907:dbl)
                    n397 = Add(x="Base line\nS2.1 (mV)", y=w906) -> (x+y=w879:dbl)
                    n398 = Subtract(x="Base line\nS2.1 (mV)", y=w906) -> (x-y=w880:dbl)
                    n399 = Subtract(x="Base line\nS2.1 (mV)", y=w907) -> (x-y=w886:dbl)
                    n400 = call "EventstoGraph (SubVI).vi"("Numerisch 2"=w887, "Array 3"=w878, "Numerisch"=w888, "Array (Eingang)"=dbl[][] [], "Numerisch 3"=w886) -> ("Array (Ausgang)"=w890:dbl[][])  [unwired: 6 in]
                    n401 = Array Max & Min(array=w877) -> (max value=w902:dbl, min value=w903:dbl)  [unwired: 2 out]
                    n402 = call "GraphLimit01.vi"("Numeric 2"=w880, "Numeric"=w879, "Array in"=w896, "Array 3"=dbl[] []) -> ("Array out"=w895:dbl[])  [unwired: 7 in]
                    n403 = Build Array("Base line\nS2.1 (mV)", "Base line\nS2.1 (mV)") -> (w899:dbl[])
                    n404 = Build Array(w902, w903) -> (w900:dbl[])
                    n405 = Build Array(w879, w880) -> (w901:dbl[])
                    n406 = Index Array(array=w890, index (col)=0 ("Index (Zeile)")) -> (element=w891:dbl[])  [unwired: 1 in]
                    n407 = Index Array(array=w890, index (col)=1 ("Index (Zeile)")) -> (element=w889:dbl[])  [unwired: 1 in]
                    n408 = Bundle(w900, w901) -> (w883:cluster{dbl[], dbl[]})  [unwired: 1 in]
                    n409 = Bundle(w900, w899) -> (w884:cluster{dbl[], dbl[]})  [unwired: 1 in]
                    n410 = Bundle(w877, "Array out"=w895) -> (w882:cluster{dbl[], "Array out":dbl[]})  [unwired: 1 in]
                    n411 = Bundle("Array (Ausgang)"=w891, "Array (Ausgang)"=w889) -> (w881:T9)  [unwired: 1 in]
                    n412 = Build Array(w884, w883, w882, w881) -> (w885:T10)
                    n413 = case shown="True" w876 {
                      tunnel: w885 -> [_ w909]
                      frame False {
                      }
                      frame True {
                        "V-SISE channel 2" <- w909
                      }
                    }
                  }
                  frame #1 {
                    n414 = Array Max & Min(array=w916) -> (max value=w925:dbl, min value=w924:dbl)  [unwired: 2 out]
                    n415 = Divide(x="Range limit\nS2.2 (mV)", y=2.0) -> (x/y=w941:dbl)
                    n416 = Divide(x="Range limit\nS2.2 (mV)", y=2.05) -> (x/y=w942:dbl)
                    n417 = Add(x="Base line \nS2.2 (mV)", y=w941) -> (x+y=w917:dbl)
                    n418 = Subtract(x="Base line \nS2.2 (mV)", y=w941) -> (x-y=w918:dbl)
                    n419 = Subtract(x="Base line \nS2.2 (mV)", y=w942) -> (x-y=w923:dbl)
                    n420 = call "EventstoGraph (SubVI).vi"("Numerisch 2"=w924, "Array 3"=w915, "Numerisch"=w925, "Array (Eingang)"=dbl[][] [], "Numerisch 3"=w923) -> ("Array (Ausgang)"=w927:dbl[][])  [unwired: 6 in]
                    n421 = Array Max & Min(array=w916) -> (max value=w937:dbl, min value=w938:dbl)  [unwired: 2 out]
                    n422 = call "GraphLimit01.vi"("Numeric 2"=w918, "Numeric"=w917, "Array in"=w914, "Array 3"=dbl[] []) -> ("Array out"=w932:dbl[])  [unwired: 7 in]
                    n423 = Build Array("Base line \nS2.2 (mV)", "Base line \nS2.2 (mV)") -> (w934:dbl[])
                    n424 = Build Array(w937, w938) -> (w935:dbl[])
                    n425 = Build Array(w917, w918) -> (w936:dbl[])
                    n426 = Index Array(array=w927, index (col)=0 ("Index (Zeile)")) -> (element=w928:dbl[])  [unwired: 1 in]
                    n427 = Index Array(array=w927, index (col)=1 ("Index (Zeile)")) -> (element=w926:dbl[])  [unwired: 1 in]
                    n428 = Bundle(w935, w936) -> (w921:cluster{dbl[], dbl[]})  [unwired: 1 in]
                    n429 = Bundle(w935, w934) -> (w922:cluster{dbl[], dbl[]})  [unwired: 1 in]
                    n430 = Bundle(w916, "Array out"=w932) -> (w920:cluster{dbl[], "Array out":dbl[]})  [unwired: 1 in]
                    n431 = Bundle("Array (Ausgang)"=w928, "Array (Ausgang)"=w926) -> (w919:T9)  [unwired: 1 in]
                    n432 = Build Array(w922, w921, w920, w919) -> (w911:T10)
                    n433 = case shown="True" w910 {
                      tunnel: w911 -> [_ w943]
                      frame False {
                      }
                      frame True {
                        "dV-SISE channel 2" <- w943
                      }
                    }
                  }
                }
              }
              frame "V channel #1" {
                n434 = Greater Or Equal?(x=w946, y=2) -> (x >= y?=w948:bool)
                n435 = And(x=w948, y=w945) -> (x .and. y?=w944:bool)
                n436 = Index Array(array=w981, index (col)=0 ("disabled index (col)")) -> (element=w950:dbl[])  [unwired: 1 in]
                n437 = Index Array(array=w981, index (col)=5 ("disabled index (col)")) -> (element=w951:dbl[])  [unwired: 1 in]
                n438 = Array Max & Min(array=w950) -> (max value=w961:dbl, min value=w960:dbl)  [unwired: 2 out]
                n439 = Divide(x="Range limit\nV1 (V)", y=2.0) -> (x/y=w978:dbl)
                n440 = Divide(x="Range limit\nV1 (V)", y=2.05) -> (x/y=w979:dbl)
                n441 = Add(x="Base line\nV1 (V)", y=w978) -> (x+y=w952:dbl)
                n442 = Subtract(x="Base line\nV1 (V)", y=w978) -> (x-y=w953:dbl)
                n443 = Subtract(x="Base line\nV1 (V)", y=w979) -> (x-y=w959:dbl)
                n444 = call "EventstoGraph (SubVI).vi"("Numerisch 2"=w960, "Array 3"=w949, "Numerisch"=w961, "Array (Eingang)"=dbl[][] [], "Numerisch 3"=w959) -> ("Array (Ausgang)"=w963:dbl[][])  [unwired: 6 in]
                n445 = Array Max & Min(array=w950) -> (max value=w974:dbl, min value=w975:dbl)  [unwired: 2 out]
                n446 = call "GraphLimit01.vi"("Numeric 2"=w953, "Numeric"=w952, "Array in"=w951, "Array 3"=dbl[] []) -> ("Array out"=w968:dbl[])  [unwired: 7 in]
                n447 = Build Array("Base line\nV1 (V)", "Base line\nV1 (V)") -> (w971:dbl[])
                n448 = Build Array(w974, w975) -> (w972:dbl[])
                n449 = Build Array(w952, w953) -> (w973:dbl[])
                n450 = Index Array(array=w963, index (col)=0 ("Index (Zeile)")) -> (element=w964:dbl[])  [unwired: 1 in]
                n451 = Index Array(array=w963, index (col)=1 ("Index (Zeile)")) -> (element=w962:dbl[])  [unwired: 1 in]
                n452 = Bundle(w972, w973) -> (w956:cluster{dbl[], dbl[]})  [unwired: 1 in]
                n453 = Bundle(w972, w971) -> (w957:cluster{dbl[], dbl[]})  [unwired: 1 in]
                n454 = Bundle(w950, "Array out"=w968) -> (w955:cluster{dbl[], "Array out":dbl[]})  [unwired: 1 in]
                n455 = Bundle("Array (Ausgang)"=w964, "Array (Ausgang)"=w962) -> (w954:T9)  [unwired: 1 in]
                n456 = Build Array(w957, w956, w955, w954) -> (w958:T10)
                n457 = case shown="True" w944 {
                  tunnel: w958 -> [_ w984]
                  frame False {
                  }
                  frame True {
                    "Voltage channel 1" <- w984
                  }
                }
              }
              frame "V channel #2" {
                n458 = Greater Or Equal?(x=w987, y=2) -> (x >= y?=w988:bool)
                n459 = And(x=w988, y=w986) -> (x .and. y?=w985:bool)
                n460 = Index Array(array=w992, index (col)=0 ("disabled index (col)")) -> (element=w990:dbl[])  [unwired: 1 in]
                n461 = Index Array(array=w992, index (col)=6 ("disabled index (col)")) -> (element=w991:dbl[])  [unwired: 1 in]
                n462 = Array Max & Min(array=w990) -> (max value=w1005:dbl, min value=w1004:dbl)  [unwired: 2 out]
                n463 = Divide(x="Range limit\nV2 (V)", y=2.0) -> (x/y=w1022:dbl)
                n464 = Divide(x="Range limit\nV2 (V)", y=2.05) -> (x/y=w1023:dbl)
                n465 = Add(x="Base line\nV2 (V)", y=w1022) -> (x+y=w996:dbl)
                n466 = Subtract(x="Base line\nV2 (V)", y=w1022) -> (x-y=w997:dbl)
                n467 = Subtract(x="Base line\nV2 (V)", y=w1023) -> (x-y=w1003:dbl)
                n468 = call "EventstoGraph (SubVI).vi"("Numerisch 2"=w1004, "Array 3"=w995, "Numerisch"=w1005, "Array (Eingang)"=dbl[][] [], "Numerisch 3"=w1003) -> ("Array (Ausgang)"=w1007:dbl[][])  [unwired: 6 in]
                n469 = Array Max & Min(array=w990) -> (max value=w1018:dbl, min value=w1019:dbl)  [unwired: 2 out]
                n470 = call "GraphLimit01.vi"("Numeric 2"=w997, "Numeric"=w996, "Array in"=w991, "Array 3"=dbl[] []) -> ("Array out"=w1012:dbl[])  [unwired: 7 in]
                n471 = Build Array("Base line\nV2 (V)", "Base line\nV2 (V)") -> (w1015:dbl[])
                n472 = Build Array(w1018, w1019) -> (w1016:dbl[])
                n473 = Build Array(w996, w997) -> (w1017:dbl[])
                n474 = Index Array(array=w1007, index (col)=0 ("Index (Zeile)")) -> (element=w1008:dbl[])  [unwired: 1 in]
                n475 = Index Array(array=w1007, index (col)=1 ("Index (Zeile)")) -> (element=w1006:dbl[])  [unwired: 1 in]
                n476 = Bundle(w1016, w1017) -> (w1000:cluster{dbl[], dbl[]})  [unwired: 1 in]
                n477 = Bundle(w1016, w1015) -> (w1001:cluster{dbl[], dbl[]})  [unwired: 1 in]
                n478 = Bundle(w990, "Array out"=w1012) -> (w999:cluster{dbl[], "Array out":dbl[]})  [unwired: 1 in]
                n479 = Bundle("Array (Ausgang)"=w1008, "Array (Ausgang)"=w1006) -> (w998:T9)  [unwired: 1 in]
                n480 = Build Array(w1001, w1000, w999, w998) -> (w1002:T10)
                n481 = case shown="True" w985 {
                  tunnel: w1002 -> [_ w1025]
                  frame False {
                  }
                  frame True {
                    "Voltage channel 2" <- w1025
                  }
                }
              }
            }
            n482 = local read "Record period (round at 5s)"() -> (w776:dbl)
            n483 = local read "Stop recording 2"() -> (w720:bool)
            n484 = Multiply(x=w776, y=10.0) -> (x*y=w780:dbl)
            n485 = Subtract(x=w780, y=10.0) -> (x-y=w778:dbl)
            n486 = Greater Or Equal?(x=w777, y=w778) -> (x >= y?=w721:bool)
            n487 = Or(x=w720, y=w721) -> (x .or. y?=w722:bool)
          }
        }
        n488 = while {
          tunnel: w546 -> [w1088]
          tunnel: w565 -> [w1106]
          tunnel: w559 -> [w1099]
          shift-right: [w1098] -> _
          shift-left: "P0: P1:" -> [w1101]
          shift-right: [w1097] -> _
          shift-left: w560 -> [w1100]
          tunnel: [w1096] -> w558
          tunnel: w557 -> [w1095]
          tunnel: [w1090] -> w519
          tunnel: [w1089] -> w518
          shift-right: [w1083] -> w551
          shift-left: w549 -> [w1081]
          shift-right: [w1082] -> w550
          shift-left: w552 -> [w1086]
          tunnel: w536 -> [w1078]
          tunnel: [w1072] -> w517
          tunnel: [w1071] -> w516
          shift-right: [w1067] -> _
          shift-left: "" -> [w1069]
          tunnel: string[] [] -> [w1070]
          tunnel: [w1068] -> _
          tunnel: w522 -> [w1064]
          tunnel: [w1063] -> w529
          i -> [w1066]
          stop <- w1062 stop-if-true
          n489 = Unbundle(w1095) -> ("task out"=w1065:refnum<k21>, "status"=w1094:bool, "code"=w1093:i32, "source"=w1092:string)
          n490 = Unbundle(w1078) -> ("refnum out"=w1074:refnum<file>, "status"=w1077:bool, "code"=w1075:i32, "source"=w1076:string)
          n491 = Divide(x=w1066, y=2) -> (x/y=w1104:dbl)
          n492 = Round Toward -Infinity(1:w1104) -> (0:w1105:dbl)
          n493 = Bundle("status"=w1094, "code"=w1093, "source"=w1092) -> (w1091:errorcluster)  [unwired: 1 in]
          n494 = Bundle("status"=w1077, "code"=w1075, "source"=w1076) -> (w1073:errorcluster)  [unwired: 1 in]
          n495 = Equal?(x=w1104, y=w1105) -> (x = y?=w1102:bool)
          n496 = while {
            tunnel: w1088 -> [w1213]
            shift-right: [w1116] -> w1062
            shift-left: FALSE -> [w1209]
            tunnel: w1106 -> [w1207]
            tunnel: w1102 -> [w1132]
            tunnel: w1066 -> [w1197]
            tunnel: w1088 -> [w1150]
            tunnel: w1088 -> [w1190]
            tunnel: w1099 -> [w1189]
            shift-right: [w1117] -> w1098
            shift-left: w1101 -> [w1192]
            shift-right: [w1188] -> w1097
            shift-left: w1100 -> [w1191]
            tunnel: [w1186] -> w1096
            tunnel: w1066 -> [w1178]
            tunnel: w1091 -> [w1176]
            tunnel: w1065 -> [w1177]
            tunnel: [w1138] -> w1090
            tunnel: [w1175] -> w1089
            tunnel: w1088 -> [w1137]
            shift-right: [w1135] -> w1080
            shift-left: dbl[][] [] -> [w1129]
            tunnel: [w1166] -> w1085
            tunnel: [w1165] -> w1084
            tunnel: w1081 -> [w1166]
            tunnel: w1086 -> [w1165]
            tunnel: w1066 -> [w1163]
            tunnel: w1074 -> [w1157]
            tunnel: w1073 -> [w1158]
            tunnel: [w1156] -> w1071
            tunnel: [w1155] -> w1072
            shift-right: [w1152] -> w1068
            shift-left: w1070 -> [w1160]
            shift-right: [w1151] -> w1067
            shift-left: w1069 -> [w1168]
            tunnel: w1066 -> [w1149]
            tunnel: w1064 -> [w1128]
            tunnel: w1064 -> [w1133]
            tunnel: [w1128] -> w1063
            i -> [w1131]
            stop <- w1211 stop-if-true
            # "Write to file"
            # "Add position / Event marks"
            # "Feed graphs"
            # "Get voltage data"
            # "Get time (s) / calculate position of probe"
            # "Control manipulator"
            # "Set graphs and controls"
            # "Set # of cycles"
            # "Stop measurement"
            n497 = disable-structure shown="Disabled" {
              disable-tunnel: w1177 -> [w1235 _]
              disable-tunnel: w1176 -> [w1234 _]
              disable-tunnel: [w1233 _] -> w1175
              disable-tunnel: [w1232 _] -> w1138
              disable-tunnel: [w1221 _] -> _
              frame Disabled {
                w1219 = 0 ("Index")
                n498 = call-poly <vilib>:"DAQmx Read.vi"("task/channels in"=w1235, "error in"=w1234) -> ("task out"=w1232:refnum<k21>, "data"=w1218:dbl[][], "error out"=w1233:errorcluster)  [unwired: 11 in]
                n499 = Index Array(array=w1218, index (row)=w1219, index (col)=w1219) -> (element=w1227:dbl)
                n500 = Index Array(array=w1218, index (row)=1 ("Index"), index (col)=w1219) -> (element=w1226:dbl)
                n501 = Index Array(array=w1218, index (row)=2 ("Index"), index (col)=w1219) -> (element=w1224:dbl)
                n502 = Index Array(array=w1218, index (row)=3 ("Index"), index (col)=w1219) -> (element=w1225:dbl)
                n503 = Divide(x=w1227, y=-0.0333) -> (x/y=w1222:dbl)
                n504 = Divide(x=w1226, y=-0.0333) -> (x/y=w1223:dbl)
                n505 = Build Array(w1222, w1223, w1224, w1225) -> (w1221:dbl[])
              }
              frame Enabled {
              }
            }
            n506 = Equal?(x=w1149, y=0) -> (x = y?=w1146:bool)
            n507 = Equal?(x=w1131, y=0) -> (x = y?=w1145:bool)
            n508 = Equal To 0?(x=w1131) -> (x = 0?=w1169:bool)
            n509 = Greater Or Equal?(x=w1163, y=2) -> (x >= y?=w1162:bool)
            "E-mark on" <- w1162
            n510 = Get Date/Time In Seconds() -> (seconds since 1Jan1904=w1208:timestamp)
            n511 = And(x=w1146, y=w1145) -> (x .and. y?=w1144:bool)
            n512 = Index Array(array=w1150, index=2) -> (element=w1195:dbl)
            n513 = Subtract(x=w1208, y=w1207) -> (x-y=w1167:dbl)
            n514 = Multiply(x=w1195, y=100.0) -> (x*y=w1194:dbl)
            n515 = Wait (ms)(milliseconds to wait=u32 10 ("Zu wartende ms")) -> ()  [unwired: 1 out]
            n516 = Index Array(array=w1213, index=2) -> (element=w1216:dbl)
            n517 = case shown="True" w1162 {
              tunnel: [FALSE "Add Mark"] -> w1161
              tunnel: w1160 -> [_ w1476]
              frame False {
              }
              frame True {
                n518 = Array Size(array=w1476) -> (size(s)=w1480:i32)
                n519 = Subtract(x=w1480, y=1) -> (x-y=w1478:i32)
                n520 = Index Array(array=w1476, index=w1478) -> (element=→"String":string)
              }
            }
            n521 = case shown="True" w1144 {
              frame False {
              }
              frame True {
                n522 = Build Array(0.0, 0.0) -> (w1469:dbl[])
                n523 = Build Array(0.0, 30.0) -> (w1470:dbl[])
                n524 = Bundle(w1470, w1469) -> (w1468:cluster{dbl[], dbl[]})  [unwired: 1 in]
                n525 = Build Array(w1468, w1468, w1468, w1468) -> (w1466:cluster{dbl[], dbl[]}[])
                n526 = local write "dV-SISE channel 1"(w1466) -> ()
                n527 = local write "deltaV SISE 1"(w1466) -> ()
                n528 = local write "deltaV SISE 2"(w1466) -> ()
                n529 = local write "V-SISE channel 1"(w1466) -> ()
                n530 = local write "V-SISE channel 2"(w1466) -> ()
                n531 = local write "dV-SISE channel 2"(w1466) -> ()
                n532 = local write "Voltage channel 1"(w1466) -> ()
                n533 = local write "Voltage channel 2"(w1466) -> ()
                n534 = local write "Enable change position 0"(FALSE) -> ()
              }
            }
            n535 = call "Feed-Position-Graph (SubVI).vi"("Array 2"=w1137, "Array"=w1129) -> ("Array 3"=→"Position probe":cluster{dbl[], dbl[]}[])  [unwired: 9 in]
            n536 = Subtract(x=w1194, y=10.0) -> (x-y=w1204:dbl)
            n537 = Subtract(x=w1194, y=20.0) -> (x-y=w1203:dbl)
            n538 = Multiply(x=w1216, y=100.0) -> (x*y=w1200:dbl)
            n539 = Build Array(0, 10, w1203, w1204) -> (w1187:dbl[])
            n540 = Equal?(x=w1197, y=0) -> (x = y?=w1123:bool)
            n541 = Add(x=1 ("y"), y=w1131) -> (x+y=w1212:i32)
            n542 = case shown="False" w1123 {
              tunnel: [w1579 w1597] -> w1122
              tunnel: w1187 -> [w1578 w1596]
              tunnel: w1131 -> [w1577 w1595]
              frame False {
                n543 = for {
                  tunnel: w1578 -> [w1586] mode=indexing
                  tunnel: w1577 -> [w1587]
                  shift-right: [w1584] -> w1579
                  shift-left: 0 -> [w1585]
                  i -> [w1582]
                  n544 = Equal?(x=w1586, y=w1587) -> (x = y?=w1583:bool)
                  n545 = case shown="True" w1583 {
                    tunnel: w1582 -> [_ w1590]
                    tunnel: [0 w1589] -> w1581
                    frame False {
                    }
                    frame True {
                      n546 = case shown="3" w1590 {
                        tunnel: [1 2 3 5] -> w1589
                        frame 0, Default {
                        }
                        frame 1 {
                        }
                        frame 2 {
                        }
                        frame 3 {
                        }
                      }
                    }
                  }
                  n547 = Add(x=w1585, y=w1581) -> (x+y=w1584:i32)
                }
              }
              frame True {
                n548 = for {
                  tunnel: w1596 -> [w1604] mode=indexing
                  tunnel: w1595 -> [w1605]
                  shift-right: [w1602] -> w1597
                  shift-left: 0 -> [w1603]
                  i -> [w1601]
                  n549 = Equal?(x=w1604, y=w1605) -> (x = y?=w1599:bool)
                  n550 = case shown="True" w1599 {
                    tunnel: w1601 -> [_ w1607]
                    tunnel: [0 w1608] -> w1600
                    frame False {
                    }
                    frame True {
                      n551 = case shown="3" w1607 {
                        tunnel: [0 0 3 4] -> w1608
                        frame 0, Default {
                        }
                        frame 1 {
                        }
                        frame 2 {
                        }
                        frame 3 {
                        }
                      }
                    }
                  }
                  n552 = Add(x=w1603, y=w1600) -> (x+y=w1602:i32)
                }
              }
            }
            n553 = Equal?(x=w1200, y=w1212) -> (x = y?=w1211:bool)
            n554 = Index Array(array=w1150, index=3 ("Index")) -> (element=w1184:dbl)
            n555 = Index Array(array=w1150, index=0 ("Index")) -> (element=w1180:dbl)
            n556 = Divide(x=w1184, y=10.0) -> (x/y=w1179:dbl)
            n557 = Greater?(x=w1179, y=w1131) -> (0:w1182:bool)
            n558 = case shown="True" w1182 {
              tunnel: w1180 -> [w1551 w1557]
              tunnel: w1131 -> [_ w1559]
              tunnel: w1132 -> [w1553 w1562]
              tunnel: w1179 -> [_ w1561]
              tunnel: [w1552 w1558] -> w1170
              tunnel: w1178 -> [_ w1556]
              frame False {
                n559 = case shown="False" w1553 {
                  tunnel: [w1554 0.0] -> w1552
                  tunnel: w1551 -> [w1554 _]
                  frame False {
                  }
                  frame True {
                  }
                }
              }
              frame True {
                n560 = Divide(x=w1557, y=w1561) -> (x/y=w1560:dbl)
                n561 = case shown="True" w1562 {
                  tunnel: w1559 -> [w1565 w1569]
                  tunnel: w1560 -> [w1564 w1573]
                  tunnel: [w1563 w1567] -> w1558
                  tunnel: w1557 -> [_ w1572]
                  tunnel: w1556 -> [_ w1566]
                  frame False {
                    n562 = Multiply(x=w1564, y=w1565) -> (x*y=w1563:dbl)
                  }
                  frame True {
                    n563 = Multiply(x=w1573, y=w1569) -> (x*y=w1574:dbl)
                    n564 = Equal?(x=w1566, y=0) -> (x = y?=w1571:bool)
                    n565 = Subtract(x=w1572, y=w1574) -> (x-y=w1568:dbl)
                    n566 = case shown="True" w1571 {
                      tunnel: [w1575 0.0] -> w1567
                      tunnel: w1568 -> [w1575 _]
                      frame False {
                      }
                      frame True {
                      }
                    }
                  }
                }
              }
            }
            n567 = case shown="\"SISE chan #1\", Default" "?" {
              selector: "?" -> [w1420 w1430 w1438 w1446]
              tunnel: w1137 -> [w1425 w1432 w1442 w1449]
              tunnel: w1129 -> [w1426 w1433 w1441 w1450]
              tunnel: w1133 -> [w1422 w1429 w1436 w1445]
              tunnel: "Start fit (% of rec. period)" -> [w1424 w1431 w1440 w1448]
              frame "SISE chan #1", Default {
                n568 = Index Array(array=w1422, index=w1420) -> (element=w1421:bool)
                n569 = call "Feed-SISE-Probe-Graph.vi"("Boolesch"=w1421, "Numerisch"=2, "Array 2"=w1426, "Array"=w1425, "Start fit (% of rec. period)"=w1424) -> ("Array 3"=→"Vprobe SISE 1":cluster{dbl[], dbl[]}[])  [unwired: 6 in]
              }
              frame "SISE chan #2" {
                n570 = Index Array(array=w1429, index=w1430) -> (element=w1428:bool)
                n571 = call "Feed-SISE-Probe-Graph.vi"("Boolesch"=w1428, "Numerisch"=3, "Array 2"=w1433, "Array"=w1432, "Start fit (% of rec. period)"=w1431) -> ("Array 3"=→"Vprobe SISE 2":cluster{dbl[], dbl[]}[])  [unwired: 6 in]
              }
              frame "V chan #1" {
                n572 = Index Array(array=w1436, index=w1438) -> (element=w1437:bool)
                n573 = call "Feed-V-Probe-Graph.vi"("Boolesch"=w1437, "Numerisch"=4, "Array 2"=w1441, "Array"=w1442, "Start fit (% of rec. period)"=w1440) -> ("Array 3"=→"Vprobe V 1":cluster{dbl[], dbl[]}[])  [unwired: 6 in]
              }
              frame "V chan #2" {
                n574 = Index Array(array=w1445, index=w1446) -> (element=w1444:bool)
                n575 = call "Feed-V-Probe-Graph.vi"("Boolesch"=w1444, "Numerisch"=5, "Array 2"=w1450, "Array"=w1449, "Start fit (% of rec. period)"=w1448) -> ("Array 3"=→"Vprobe V 2":cluster{dbl[], dbl[]}[])  [unwired: 6 in]
              }
            }
            n576 = disable-structure shown="Disabled" {
              disable-tunnel: w1192 -> [w1244 _]
              disable-tunnel: w1191 -> [w1243 _]
              disable-tunnel: w1190 -> [w1242 _]
              disable-tunnel: w1189 -> [w1241 _]
              disable-tunnel: [w1240 _] -> w1188
              disable-tunnel: [w1239 _] -> w1186
              disable-tunnel: w1132 -> [w1238 _]
              disable-tunnel: w1122 -> [w1237 _]
              disable-tunnel: [w1236 _] -> w1117
              frame Disabled {
                n577 = case shown="1" w1237 {
                  tunnel: w1241 -> [w1245 w1258 w1302 w1309 w1321 w1368]
                  tunnel: w1243 -> [w1247 w1265 w1305 w1308 w1320 w1367]
                  tunnel: [w1247 w1265 w1305 w1308 w1319 w1366] -> w1240
                  tunnel: w1242 -> [_ w1264 _ _ _ _]
                  tunnel: w1238 -> [_ w1252 _ _ w1313 w1360]
                  tunnel: w1244 -> [w1246 w1251 w1301 w1307 w1316 w1363]
                  tunnel: [w1246 w1251 w1301 w1307 w1317 w1364] -> w1236
                  tunnel: [w1245 w1250 w1300 w1306 w1314 w1361] -> w1239
                  frame 0, Default {
                  }
                  frame 1 {
                    n578 = local read "left"() -> (w1249:bool)
                    n579 = Index Array(array=w1264, index=0) -> (element=w1266:dbl)
                    n580 = Index Array(array=w1264, index=1) -> (element=w1257:dbl)
                    n581 = Cosine(x=w1257) -> (cos(x)=w1256:dbl)
                    n582 = Sine(x=w1257) -> (sin(x)=w1255:dbl)
                    n583 = case shown="False" w1249 {
                      tunnel: [10.0 -10.0] -> w1248
                      frame False {
                      }
                      frame True {
                      }
                    }
                    n584 = Multiply(x=w1266, y=w1256) -> (x*y=w1263:dbl)
                    n585 = Multiply(x=w1266, y=w1255) -> (x*y=w1262:dbl)
                    n586 = Multiply(x=w1263, y=w1248) -> (x*y=w1260:dbl)
                    n587 = Multiply(x=w1262, y=10.0) -> (x*y=w1261:dbl)
                    n588 = for {
                      tunnel: w1265 -> [w1280] mode=indexing
                      tunnel: w1260 -> [w1282]
                      tunnel: w1261 -> [w1281]
                      shift-right: [w1276] -> w1254
                      shift-left: "ABS " -> [w1278]
                      tunnel: w1252 -> [w1271]
                      i -> [w1273]
                      n589 = case shown="True" w1271 {
                        tunnel: w1273 -> [w1283 _]
                        tunnel: [w1283 1] -> w1272
                        frame False {
                        }
                        frame True {
                        }
                      }
                      n590 = case shown="1" w1272 {
                        tunnel: w1282 -> [w1294 _ _]
                        tunnel: w1281 -> [_ _ w1298]
                        tunnel: w1280 -> [w1295 w1296 w1299]
                        tunnel: [w1293 w1296 w1297] -> w1279
                        frame 0, Default {
                          n591 = Add(x=w1295, y=w1294) -> (x+y=w1293:dbl)
                        }
                        frame 1 {
                        }
                        frame 2 {
                          n592 = Add(x=w1299, y=w1298) -> (x+y=w1297:dbl)
                        }
                      }
                      n593 = Number To Decimal String(number=w1279) -> (decimal integer string=w1277:string)  [unwired: 1 in]
                      n594 = Equal?(x=2, y=w1273) -> (x = y?=w1274:bool)
                      n595 = case shown="True" w1274 {
                        tunnel: w1278 -> [w1288 w1292]
                        tunnel: w1277 -> [w1287 w1290]
                        tunnel: [w1285 w1291] -> w1276
                        frame False {
                          n596 = Concatenate Strings(w1288, w1287, "\t") -> (w1285:string)
                        }
                        frame True {
                          n597 = Concatenate Strings(w1292, w1290, "\r\n") -> (w1291:string)
                        }
                      }
                    }
                    n598 = VISA Write(VISA resource name=w1258, write buffer=w1254) -> (VISA resource name out=w1250:refnum<visa-resource-name>)  [unwired: 1 in, 2 out]
                  }
                  frame 2 {
                    n599 = property class="Instr"(reference=w1302) -> (reference out=w1303:refnum<visa-resource-name>, "Bytes at Port"=w1304:u32)  [unwired: 1 in, 1 out]
                    n600 = VISA Read(VISA resource name=w1303, byte count=w1304) -> (VISA resource name out=w1300:refnum<visa-resource-name>)  [unwired: 1 in, 3 out]
                  }
                  frame 3 {
                    n601 = Concatenate Strings("POS", "\r\n") -> (w1312:string)
                    n602 = VISA Write(VISA resource name=w1309, write buffer=w1312) -> (VISA resource name out=w1306:refnum<visa-resource-name>)  [unwired: 1 in, 2 out]
                  }
                  frame 4 {
                    n603 = property class="Instr"(reference=w1321) -> (reference out=w1323:refnum<visa-resource-name>, "Bytes at Port"=w1322:u32)  [unwired: 1 in, 1 out]
                    n604 = VISA Read(VISA resource name=w1323, byte count=w1322) -> (VISA resource name out=w1315:refnum<visa-resource-name>, read buffer=w1318:string)  [unwired: 1 in, 2 out]
                    n605 = case shown="True" w1313 {
                      tunnel: w1320 -> [w1339 w1358]
                      tunnel: [w1339 w1357] -> w1319
                      tunnel: w1318 -> [w1328 w1343]
                      tunnel: [w1333 w1352] -> w1317
                      tunnel: w1316 -> [w1332 w1351]
                      tunnel: w1315 -> [w1324 w1342]
                      tunnel: [w1324 w1342] -> w1314
                      frame False {
                        n606 = Match Pattern(string=w1332, regular expression="P0:") -> (match substring=w1337:string, after substring=w1336:string)  [unwired: 1 in, 2 out]
                        n607 = String Length(string=w1328) -> (length=w1331:i32)
                        n608 = Match Pattern(string=w1336, regular expression="P1:") -> (before substring=w1325:string, match substring=w1338:string)  [unwired: 1 in, 2 out]
                        n609 = Subtract(x=w1331, y=1) -> (x-y=w1329:i32)
                        n610 = String Subset(string=w1328, length (rest)=w1329) -> (substring=w1327:string)  [unwired: 1 in]
                        n611 = Concatenate Strings(w1337, w1325, w1338, w1327, "\t") -> (w1333:string)
                      }
                      frame True {
                        n612 = Match Pattern(string=w1351, regular expression="P0:") -> (match substring=w1353:string, after substring=w1355:string)  [unwired: 1 in, 2 out]
                        n613 = String Length(string=w1343) -> (length=w1350:i32)
                        n614 = Subtract(x=w1350, y=1) -> (x-y=w1348:i32)
                        n615 = Match Pattern(string=w1355, regular expression="P1:") -> (match substring=w1345:string, after substring=w1346:string)  [unwired: 1 in, 2 out]
                        n616 = String Subset(string=w1343, length (rest)=w1348) -> (substring=w1347:string)  [unwired: 1 in]
                        n617 = Concatenate Strings(w1353, w1347, "\t", w1345, w1346) -> (w1352:string)
                        n618 = call "GetAxisValuesI (SubVI).vi"("read buffer"=w1343) -> ("Array"=w1340:dbl[])  [unwired: 10 in]
                        n619 = Replace Array Subset(array=w1358, new element=w1340, index=0 ("Index")) -> (w1357:dbl[])
                      }
                    }
                  }
                  frame 5 {
                    n620 = property class="Instr"(reference=w1368) -> (reference out=w1370:refnum<visa-resource-name>, "Bytes at Port"=w1369:u32)  [unwired: 1 in, 1 out]
                    n621 = VISA Read(VISA resource name=w1370, byte count=w1369) -> (VISA resource name out=w1362:refnum<visa-resource-name>, read buffer=w1365:string)  [unwired: 1 in, 2 out]
                    n622 = case shown="True" w1360 {
                      tunnel: w1367 -> [w1386 w1405]
                      tunnel: [w1386 w1404] -> w1366
                      tunnel: w1365 -> [w1375 w1390]
                      tunnel: [w1380 w1399] -> w1364
                      tunnel: w1363 -> [w1379 w1398]
                      tunnel: w1362 -> [w1371 w1388]
                      tunnel: [w1371 w1387] -> w1361
                      tunnel: "Enable change position 0" -> [_ w1389]
                      frame False {
                        n623 = Match Pattern(string=w1379, regular expression="P0:") -> (match substring=w1384:string, after substring=w1383:string)  [unwired: 1 in, 2 out]
                        n624 = String Length(string=w1375) -> (length=w1378:i32)
                        n625 = Match Pattern(string=w1383, regular expression="P1:") -> (before substring=w1372:string, match substring=w1385:string)  [unwired: 1 in, 2 out]
                        n626 = Subtract(x=w1378, y=1) -> (x-y=w1376:i32)
                        n627 = String Subset(string=w1375, length (rest)=w1376) -> (substring=w1374:string)  [unwired: 1 in]
                        n628 = Concatenate Strings(w1384, w1372, w1385, w1374, "\t") -> (w1380:string)
                      }
                      frame True {
                        n629 = Match Pattern(string=w1398, regular expression="P0:") -> (match substring=w1400:string, after substring=w1402:string)  [unwired: 1 in, 2 out]
                        n630 = String Length(string=w1390) -> (length=w1397:i32)
                        n631 = Subtract(x=w1397, y=1) -> (x-y=w1395:i32)
                        n632 = Match Pattern(string=w1402, regular expression="P1:") -> (match substring=w1392:string, after substring=w1393:string)  [unwired: 1 in, 2 out]
                        n633 = String Subset(string=w1390, length (rest)=w1395) -> (substring=w1394:string)  [unwired: 1 in]
                        n634 = case shown="False" w1389 {
                          tunnel: w1405 -> [w1407 w1413]
                          tunnel: [w1407 w1412] -> w1404
                          tunnel: w1390 -> [_ w1411]
                          tunnel: w1388 -> [w1406 w1408]
                          tunnel: [w1406 w1408] -> w1387
                          frame False {
                          }
                          frame True {
                            n635 = call "GetAxisValuesI (SubVI).vi"("read buffer"=w1411) -> ("Array"=w1409:dbl[])  [unwired: 10 in]
                            n636 = Replace Array Subset(array=w1413, new element=w1409, index=0 ("Index")) -> (w1412:dbl[])
                          }
                        }
                        n637 = Concatenate Strings(w1400, w1394, "\t", w1392, w1393) -> (w1399:string)
                      }
                    }
                  }
                }
              }
              frame Enabled {
              }
            }
            n638 = case shown="True" w1169 {
              tunnel: w1117 -> [_ w1502]
              tunnel: [w1486 w1502] -> w1153
              tunnel: w1161 -> [w1487 _]
              tunnel: w1160 -> [w1482 w1511]
              tunnel: w1167 -> [w1485 w1510]
              tunnel: [w1484 w1502] -> w1151
              tunnel: w1168 -> [w1484 w1503]
              tunnel: [w1483 w1509] -> w1152
              frame False {
                n639 = case shown="True" w1487 {
                  tunnel: ["" "Event Mark"] -> w1486
                  tunnel: w1485 -> [_ w1501]
                  tunnel: w1482 -> [w1489 w1494]
                  tunnel: [w1489 w1495] -> w1483
                  frame False {
                  }
                  frame True {
                    n640 = Divide(x=w1501, y=60.0) -> (x/y=w1499:dbl)
                    n641 = Number To Fractional String(number=w1499, precision (6)=i16 2 ("Genauigkeit (6)")) -> (F-format string=w1497:string)  [unwired: 2 in]
                    n642 = Concatenate Strings(w1497, " min: ", "\t", "Event Mark", "\t") -> (w1493:string)
                    n643 = Insert Into Array(array=w1494, new element=w1493) -> (w1495:string[])  [unwired: 1 in]
                  }
                }
              }
              frame True {
                n644 = Match Pattern(string=w1502, regular expression="P1:") -> (before substring=w1506:string)  [unwired: 1 in, 3 out]
                n645 = Match Pattern(string=w1503, regular expression="P1:") -> (before substring=w1504:string)  [unwired: 1 in, 3 out]
                n646 = Not Equal?(x=w1506, y=w1504) -> (x != y?=w1508:bool)
                n647 = case shown="True" w1508 {
                  tunnel: w1511 -> [w1512 w1534]
                  tunnel: [w1512 w1535] -> w1509
                  tunnel: w1502 -> [_ w1523]
                  tunnel: w1503 -> [_ w1522]
                  tunnel: w1510 -> [_ w1520]
                  frame False {
                  }
                  frame True {
                    n648 = Divide(x=w1520, y=60.0) -> (x/y=w1518:dbl)
                    n649 = Match Pattern(string=w1523, regular expression="P0:") -> (after substring=w1533:string)  [unwired: 1 in, 3 out]
                    n650 = Number To Fractional String(number=w1518, precision (6)=i16 2) -> (F-format string=w1514:string)  [unwired: 2 in]
                    n651 = Match Pattern(string=w1522, regular expression="P0:") -> (after substring=w1528:string)  [unwired: 1 in, 3 out]
                    n652 = Match Pattern(string=w1533, regular expression="P1:") -> (before substring=w1532:string)  [unwired: 1 in, 3 out]
                    n653 = Match Pattern(string=w1528, regular expression="P1:") -> (before substring=w1527:string)  [unwired: 1 in, 3 out]
                    n654 = Concatenate Strings(w1514, "\t", "min: Move ") -> (w1517:string)
                    n655 = call "GetAxisValuesII (SubVI).vi"("read buffer"=w1532) -> ("Array"=w1529:dbl[])  [unwired: 10 in]
                    n656 = call "GetAxisValuesII (SubVI).vi"("read buffer"=w1527) -> ("Array"=w1524:dbl[])  [unwired: 10 in]
                    n657 = for {
                      tunnel: w1529 -> [w1545] mode=indexing
                      tunnel: w1524 -> [w1544] mode=indexing
                      shift-right: [w1546] -> w1515
                      shift-left: w1517 -> [w1547]
                      i -> [w1542]
                      n658 = Subtract(x=w1545, y=w1544) -> (x-y=w1539:dbl)
                      n659 = Divide(x=w1539, y=10.0) -> (x/y=w1541:dbl)
                      n660 = case shown="0, Default" w1542 {
                        tunnel: ["X " "Y " "Z "] -> w1538
                        frame 0, Default {
                        }
                        frame 1 {
                        }
                        frame 2 {
                        }
                      }
                      n661 = Number To Fractional String(number=w1541, precision (6)=i16 2 ("Genauigkeit (6)")) -> (F-format string=w1537:string)  [unwired: 2 in]
                      n662 = Concatenate Strings(w1547, w1538, w1537, "\t") -> (w1546:string)
                    }
                    n663 = Insert Into Array(array=w1534, new element=w1515) -> (w1535:string[])  [unwired: 1 in]
                  }
                }
              }
            }
            n664 = call "EsingleGenerator.vi"("Numeric in"=w1131, "Boolean"=w1132) -> ("Numeric out"=w1111:dbl)  [unwired: 9 in]
            n665 = Build Array(w1167, w1170) -> (w1118:dbl[])
            n666 = Multiply(x=w1111, y="V SISE\nch #1") -> (x*y=w1114:dbl)
            n667 = Multiply(x=w1111, y="V SISE\nch #2") -> (x*y=w1113:dbl)
            n668 = Random Number (0-1)() -> (number: 0 to 1=w1143:dbl)
            n669 = Random Number (0-1)() -> (number: 0 to 1=w1174:dbl)
            n670 = Add(x=w1113, y=8.0) -> (x+y=w1142:dbl)
            n671 = Add(x=w1114, y=6.0) -> (x+y=w1173:dbl)
            n672 = Add(x=w1142, y=w1143) -> (x+y=w1139:dbl)
            n673 = Add(x=w1173, y=w1174) -> (x+y=w1140:dbl)
            n674 = case shown="False" "Stop measurent" {
              tunnel: [w1613 TRUE] -> w1116
              tunnel: w1209 -> [w1613 _]
              frame False {
              }
              frame True {
              }
            }
            "Stop recording" <- w1116
            n675 = Build Array(w1140, w1139, "Vch #1", "Vch\n#2") -> (w1108:dbl[])
            n676 = for {
              tunnel: w1108 -> [w1453] mode=indexing
              tunnel: w1128 -> [w1456] mode=indexing
              shift-right: [w1454] -> w1127
              shift-left: dbl[] [] -> [w1455]
              shift-right: [w1451] -> w1119
              shift-left: dbl[] [] -> [w1452]
              n677 = case shown="False" w1456 {
                tunnel: w1455 -> [w1460 w1465]
                tunnel: [w1460 w1464] -> w1454
                tunnel: w1453 -> [_ w1461]
                tunnel: w1452 -> [w1459 w1463]
                tunnel: [w1458 w1462] -> w1451
                frame False {
                  n678 = Insert Into Array(array=w1459, new element=0.0 ("Neues Element/Teil-Array")) -> (w1458:dbl[])  [unwired: 1 in]
                }
                frame True {
                  n679 = Insert Into Array(array=w1465, new element=w1461) -> (w1464:dbl[])  [unwired: 1 in]
                  n680 = Insert Into Array(array=w1463, new element=w1461) -> (w1462:dbl[])  [unwired: 1 in]
                }
              }
            }
            n681 = Insert Into Array(array=w1118, new element=w1119) -> (w1120:dbl[])  [unwired: 1 in]
            n682 = Insert Into Array(array=w1118, new element=w1127) -> (w1125:dbl[])  [unwired: 1 in]
            n683 = for {
              tunnel: w1125 -> [w1416] mode=indexing
              shift-right: [w1415] -> w1124
              shift-left: "" -> [w1417]
              n684 = Number To Fractional String(number=w1416) -> (F-format string=w1418:string)  [unwired: 3 in]
              n685 = Concatenate Strings(w1417, w1418, "\t") -> (w1415:string)
            }
            n686 = Insert Into Array(array=w1129, new element=w1120) -> (w1135:dbl[][])  [unwired: 2 in]
            n687 = Concatenate Strings(w1124, w1153, "\r\n") -> (w1154:string)
            n688 = Write to Text File(file (use dialog)=w1157, text=w1154, error in=w1158) -> (refnum out=w1156:refnum<file>, error out=w1155:errorcluster)  [unwired: 1 in, 1 out]
          }
          "Stop recording 2" <- w1062
          n689 = Bundle(w1068, w1080) -> (w1079:cluster{string[], dbl[][]})  [unwired: 1 in]
          n690 = Enqueue Element(queue=w1085, element=w1079, error in (no error)=w1084) -> (queue out=w1083:refnum<queue>, error out=w1082:errorcluster)  [unwired: 1 in, 1 out]
        }
        n691 = Unbundle(w518) -> ("status"=w556:bool, "code"=w555:i32, "source"=w554:string)
        n692 = call <vilib>:"DAQmx Stop Task.vi"("task/channels in"=w519, "error in"=w518) -> ()  [unwired: 12 in, 2 out]
        n693 = Close File(refnum=w516, error in=w517) -> ()  [unwired: 2 out]
        n694 = Unbundle(w517) -> ("status"=w535:bool, "code"=w534:i32, "source"=w533:string)
        n695 = Bundle("task out"=w519, "status"=w556, "code"=w555, "source"=w554) -> (w553:T5)  [unwired: 1 in]
        n696 = Bundle("refnum out"=w516, "status"=w535, "code"=w534, "source"=w533) -> (w532:T4)  [unwired: 1 in]
        n697 = Release Queue(queue=w551, error in (no error)=w550) -> ()  [unwired: 1 in, 3 out]
      }
      frame 2 {
        n698 = while {
          tunnel: w1617 -> [w1625]
          tunnel: [w1624] -> w1616
          stop <- w1628 stop-if-true
          n699 = Wait (ms)(milliseconds to wait=u32 100 ("Zu wartende ms")) -> ()  [unwired: 1 out]
          n700 = case shown="True" "Stop programm" {
            tunnel: w1625 -> [w1630 _]
            tunnel: [w1630 TRUE] -> w1624
            frame False {
            }
            frame True {
            }
          }
          n701 = Or(x="New measurement", y="Stop programm") -> (x .or. y?=w1628:bool)
        }
      }
    }
    "Registerkarte" <- w27
  }
